vi "MotorControlMina.vi"() -> ()   [LabVIEW 2014]
uses:
  <vilib>/Utility/error.llb/DialogType.ctl
  <vilib>/Analysis/baseanly.llb/Mean (DBL).vi
  <vilib>/DAQmx/create/channels.llb/DAQmx Create Channel (DO-Digital Output).vi
  <vilib>/DAQmx/read.llb/DAQmx Read (Digital Bool 1Line 1Point).vi
  <vilib>/Utility/inputDevices.llb/joystickAcquire.vi
  <vilib>/Utility/inputDevices.llb/closeJoystick.vi
  <vilib>/DAQmx/create/channels.llb/DAQmx Create Channel (AI-Voltage-Basic).vi
  <vilib>/DAQmx/configure/timing.llb/DAQmx Timing (Sample Clock).vi
  <vilib>/DAQmx/read.llb/DAQmx Read (Analog 2D DBL NChan NSamp).vi
  <vilib>/DAQmx/create/channels.llb/DAQmx Create Channel (AO-Voltage-Basic).vi
  <vilib>/DAQmx/write.llb/DAQmx Write (Analog DBL 1Chan 1Samp).vi
  <vilib>/DAQmx/write.llb/DAQmx Write (Digital Bool 1Line 1Point).vi
  <vilib>/Analysis/NI_AALBase.lvlib
panel:
  in  "Offset (V)":dbl=5.0
  out "Oscillate Mirror? 2":bool
  out "Mirror Voltage":dbl
  in  "Oscillate Mirror?":bool
  in  "Period (s)":i32=1
  in  "Amplitude (V)":dbl=4.0
  in  "Stop":bool
  in  "ForceExtInitConst":dbl[](array[numeric])
  out "InstrumentMode":T1(ring)=enum."Shutdown"
  in  "XMotorRef":refnum<k7>(container)
  in  "YMotorRef":refnum<k7>(container)
  in  "ZMotorRef":refnum<k7>(container)
  out "JoystOffset":T2={"XOffset"=-99999, "YOffset"=-99999, "ZOffset"=-99999}
  out "RelJoyPos":T3
  in  "InterfaceSelector":T4(tab)
  in  "GoToTopDisp":bool
  in  "GoToBottDisp":bool
  in  "GoToExpLoc":bool
  in  "SaveTopDisp":bool
  in  "SaveBottDisp":bool
  in  "SaveExpLoc":bool
  out "Top Dispenser":T5={"X Pos (mm)"=0.5532008, "Y Pos (mm)"=0.030929338, "Z Pos (mm)"=0.77973413} {"Y Pos (mm)" format="%.3f"; "Z Pos (mm)" format="%.3f"; "X Pos (mm)" format="%.3f"}
  out "Bottom Dispenser":T5={"X Pos (mm)"=0.600309, "Y Pos (mm)"=-1.1540928, "Z Pos (mm)"=0.7938141} {"Y Pos (mm)" format="%.3f"; "Z Pos (mm)" format="%.3f"; "X Pos (mm)" format="%.3f"}
  out "Experiment Region":T5={"X Pos (mm)"=1.4278219, "Y Pos (mm)"=-0.74810517, "Z Pos (mm)"=0.7938141} {"Y Pos (mm)" format="%.3f"; "Z Pos (mm)" format="%.3f"; "X Pos (mm)" format="%.3f"}
  in  "PreviewPanel":T6(tab)
  out "Diagnostic Display":cluster{dbl, dbl}(graph)={100.78259213882863, 10.649843481998925}
  out "VertReading":dbl=0.0051513671875 format="%.3f"
  out "HorizReading":dbl=0.00535888671875 format="%.3f"
  out "QPD B \n(Steerable Trap)":T7={"Horizontal Voltage (V)"=-0.009930419921875, "Vertical Voltage (V)"=-0.077978515625, "Sum Voltage (V)"=-0.056793212890625, "Horizontal Signal (NormV)"=0.17485222998387961, "Vertical Signal (NormV)"=1.3730252552391187} {"Vertical Signal (NormV)" format="%.4f"; "Horizontal Signal (NormV)" format="%#.4f"; "Sum Voltage (V)" format="%.4f"; "Vertical Voltage (V)" format="%.4f"; "Horizontal Voltage (V)" format="%.4f"}
  out "QPD A \n(Fixed Trap)":T7={"Horizontal Voltage (V)"=-0.151220703125, "Vertical Voltage (V)"=-0.02420654296875, "Sum Voltage (V)"=-0.1012939453125, "Horizontal Signal (NormV)"=1.4928898529766208, "Vertical Signal (NormV)"=0.23897324656543747} {"Vertical Signal (NormV)" format="%.4f"; "Horizontal Signal (NormV)" format="%.4f"; "Sum Voltage (V)" format="%.4f"; "Vertical Voltage (V)" format="%.4f"; "Horizontal Voltage (V)" format="%.4f"}
  in  "PreviewDataAcquision":T8={"Sampling Freq (Hz)"=2500.0, "#Samples Averaged"=50}
  in  "Trap A (Steerable)  Params":T9={"X Stiff. (pN/nm)"=0.056, "X Alpha (nm/NV)"=976.0, "X Offset (NV)"=-0.02, "Y Stiff. (pN/nm)"=0.056, "Y Alpha (nm/NV)"=976.0, "Y Offset (NV)"=0.008}
  in  "Trap B (Fixed)  Params":T9={"X Stiff. (pN/nm)"=0.063, "X Alpha (nm/NV)"=1056.0, "X Offset (NV)"=-0.022, "Y Stiff. (pN/nm)"=0.063, "Y Alpha (nm/NV)"=1056.0, "Y Offset (NV)"=-0.013}
  in  "Z Motor Settings":T10={"Joyst Min Signal"=10.0, "Joyst Max Signal"=30000.0, "Vmax (mm/s)"=0.005, "Acc (mm/s/s)"=0.2, "+ JoystDirection"=2, "- JoystDirection"=1} {"Acc (mm/s/s)" format="%#.3f"; "Vmax (mm/s)" format="%#.3f"}
  in  "Y Motor Settings":T10={"Joyst Min Signal"=10.0, "Joyst Max Signal"=20000.0, "Vmax (mm/s)"=0.03, "Acc (mm/s/s)"=0.5, "+ JoystDirection"=1, "- JoystDirection"=2} {"Acc (mm/s/s)" format="%#.3f"; "Vmax (mm/s)" format="%#.3f"}
  in  "X Motor Settings":T10={"Joyst Min Signal"=10.0, "Joyst Max Signal"=20000.0, "Vmax (mm/s)"=0.03, "Acc (mm/s/s)"=0.5, "+ JoystDirection"=2, "- JoystDirection"=1} {"Acc (mm/s/s)" format="%#.3f"; "Vmax (mm/s)" format="%#.3f"}
  in  "Motor Cruise Param":T11={"X Acc (mm/s^2)"=0.3, "X Vmax (mm/s)"=0.3, "Y Acc (mm/s^2)"=0.3, "Y Vmax (mm/s)"=0.3, "Z Acc (mm/s^2)"=0.1, "Z Vmax (mm/s)"=0.1}
  in  "Motor Limits":T12={"XMin"=-0.8, "XMax"=3.0, "YMin"=-2.0, "YMax"=2.0, "ZMin"=0.0, "ZMax"=2.0}
  in  "Steerable Mirror Calibration":T13={"Hor. Scaling (nm/V)"=760.0, "Vert. Scaling (nm/V)"=760.0, "Hor. Mirr. Offset (V)"=0.0, "Vert. Mirr. Offset (V)"=0.0}
  in  "SampRate/Ch":dbl=25000.0
  in  "AveragingWindow":i32=10
  in  "Steerable \nTrap\n(F12)":bool
  in  "Fixed\nTrap\n(F11)":bool
  in  "BMHorizSlider(V)":dbl(slide)=0.0059356689453125 scale=0.0..10.0
  in  "BMSliderVert(V)":dbl(slide)=0.005126953125 scale=0.0..10.0 scale format="%#_3f"
  in  "Align Traps Vertically":bool
  in  "MaxHorizontalTrapSeparation":bool
  out "X Motor State":T14={"Direction"=0, "Vel (mm/s)"=0.0, "IsActive?"=FALSE, "Pos (mm)"=-0.2957381} {"Pos (mm)" format="%#.3f"; "Vel (mm/s)" format="%#.4f"}
  out "Y Motor State":T14={"Direction"=0, "Vel (mm/s)"=0.0, "IsActive?"=FALSE, "Pos (mm)"=0.016441232} {"Pos (mm)" format="%#.3f"; "Vel (mm/s)" format="%#.4f"}
  out "Z Motor State":T14={"Direction"=0, "Vel (mm/s)"=0.0, "IsActive?"=FALSE, "Pos (mm)"=-0.26253498} {"Pos (mm)" format="%#.3f"; "Vel (mm/s)" format="%#.4f"}
  out "Move Z":bool
  out "Move XY":bool
  in  "MotorLoopDelay":u32=100
  out "Waveform Chart":T15(graph)={"[0]"=0.0023651123, "[1]"=0.0025787354, "[2]"=0.0019226074, "[3]"=0.0018310547, "[4]"=0.006378174, "[5]"=0.004486084, "[6]"=0.0008239746, "[7]"=0.0034179688}
  in  "StopPassiveMode":bool caption="stop"
  out "LowFreqFilePath":string="C:\\Data\\091813\\091813N02.psv"
  in  "PMVertSlider(V)":dbl(slide)=0.005145263671875 scale=0.0..10.0 scale format="%#_3f"
  in  "PMHorizSlider(V)":dbl(slide)=0.0045623779296875 scale=2.0..10.0
  out "IsPassiveModeActive?":bool caption="stop"
  out "Force TrapA":cluster{"x":dbl[], "y":dbl[]}[](graph)
  out "Noise-Ext":cluster{"x":dbl[], "y":dbl[]}[](graph)
  out "Force TrapB":cluster{"x":dbl[], "y":dbl[]}[](graph)
  out "OffsetFilePath":string="C:\\Data\\091813\\091813N08.ofs"
  in  "InitialConst":dbl[](array[numeric])
  in  "Stop Voltage (V)":dbl=4.0
  out "OM Vert MTA Voltage":dbl=0.0042724609375 format="%#.3f"
  out "OM Horiz MTA Voltage":dbl format="%#.3f"
  in  "HorizMirrCalib(nm/V)":dbl=752.0
  in  "HorizMirrOffs(V)":dbl
  in  "ClearChart":bool
  in  "Step (V)":dbl=0.01
  in  "#PtsToWait":i32=100
  in  "VertMirrOffs(V)":dbl
  in  "VertMirrCalib(nm/V)":dbl=752.0
  out "IsOffsetModeActive?":bool caption="stop"
  in  "StopOffset":bool caption="stop"
  out "ProgressBar":i32(slide)=200 min=0 max=512 step=1 scale=0.0..200.0
  in  "WindowSample#":i32=2048
  out "HiFreqDiagnostic":T16(graph)={"[0]"=0.002342537045478821, "[1]"=0.0025282055139541626, "[2]"=0.0019662082195281982, "[3]"=0.0019291043281555176, "[4]"=0.005142837762832642, "[5]"=0.0045330822467803955, "[6]"=0.0008034706115722656, "[7]"=0.0034596025943756104}
  in  "HiFSamplingRate/Ch":dbl=25000.0
  out "File Name and Path":string="C:\\Data\\091813\\091813N01.brw"
  in  "Total#OfWindows":dbl=200.0
  out "IsForceExtActive?":bool=TRUE
  in  "FEX Axis":bool=TRUE
  out "ForceExtensionFilePath":string="C:\\Data\\091813\\091813N00.pul"
  in  "StopForceExtension":bool caption="stop"
  in  "#FEXPtsToWait":i32=500
  in  "Mirror Step (V)":dbl=0.0020000000949949026
  out "FEX Force TrapA":cluster{"x":dbl[], "y":dbl[]}[](graph)
  out "FEX Noise-Ext":cluster{"x":dbl[], "y":dbl[]}[](graph)
  in  "Direction":bool=TRUE
  in  "IsPullActive?":bool
  in  "Clear FEX Chart":bool
  in  "FEX HorizMirrOffs(V)":dbl
  in  "FEX HorizMirrCalib(nm/V)":dbl=752.0
  out "FEX Mirror Y Volt":dbl=0.00537109375 format="%#.3f"
  out "FEX Mirror X Volt":dbl=0.004638671875 format="%#.3f"
  # "ClpXP Optical Tweezers"
  # "Chamber Locations"
  # "Need a Button Here that would read the \nNormalized Offset and save it"
  # "Off"
  # "On"
  # "Off"
  # "On"
  # "Thorlabs Motor Status"
  # "Passive Mode"
  # "when I switch tabs from the passive mode to basic mode, the recording doesn't stop"
  # "The sliders don't do anything in passive mode, fix it"
  # "Whenever I click on Ackquire Offset, it goes back to the basic operation, then I have to ckick again"
  # "Trap Motion Control"
  # "Steerable Mirror Info"
  # "Zero-Force Offset Mode"
  # "High Frequency Data Acquisition"
  # "Adjust the length of acquisition time"
  # "Force-Extension Mode"
  # "Y"
  # "+"
  # "X"
  # "-"
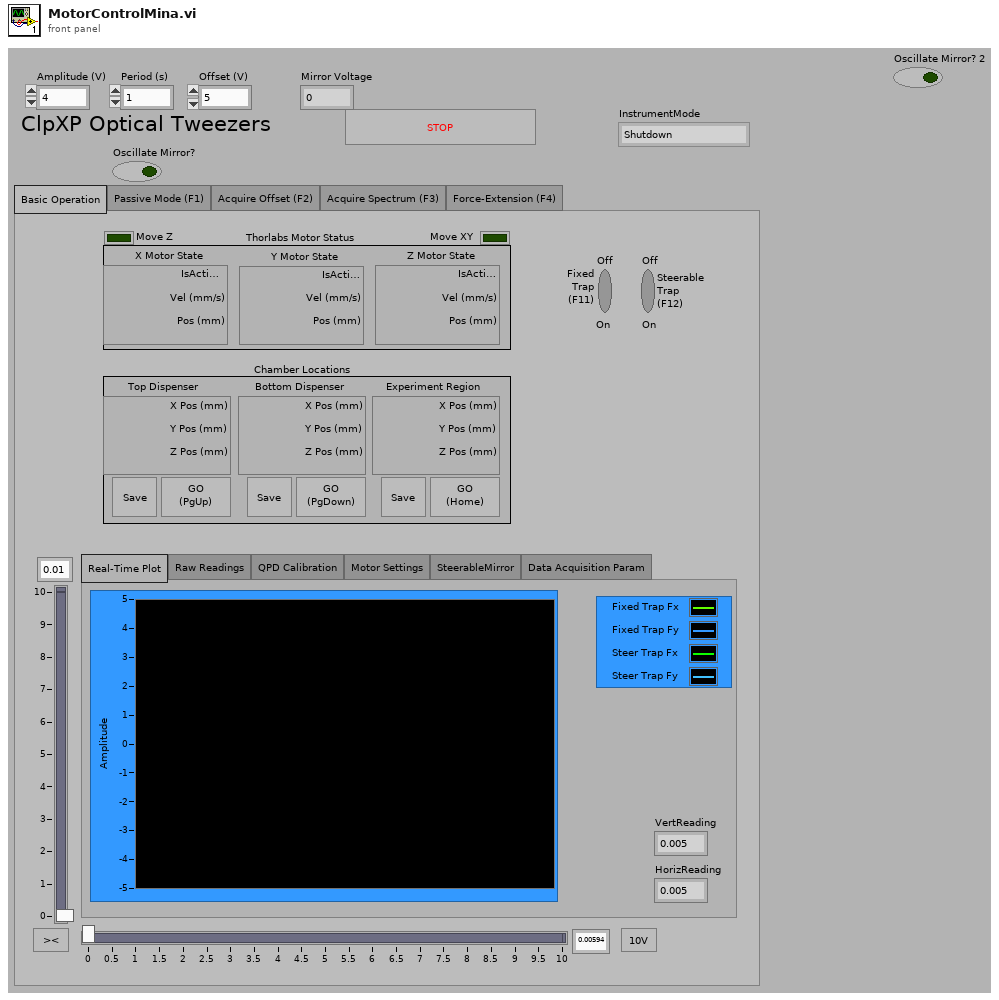
[diagram p1: front panel]
types:
  T1 = enum16{"InitializeJoystick", "InitializeMotors", "BasicMode", "PassiveMode", "AcquireOffsetMode", "AcquireSpectrumMode", "Force-ExtensionMode", "Shutdown"}
  T2 = cluster{"XOffset":i32, "YOffset":i32, "ZOffset":i32}
  T3 = cluster{"XRelPos":i32, "YRelPos":i32, "ZRelPos":i32}
  T4 = enum32{"Basic Operation", "Passive Mode (F1)", "Acquire Offset (F2)", "Acquire Spectrum (F3)", "Force-Extension (F4)"}
  T5 = cluster{"X Pos (mm)":sgl, "Y Pos (mm)":sgl, "Z Pos (mm)":sgl}
  T6 = enum32{"Real-Time Plot", "Raw Readings", "QPD Calibration", "Motor Settings", "SteerableMirror", "Data Acquisition Param"}
  T7 = cluster{"Horizontal Voltage (V)":dbl, "Vertical Voltage (V)":dbl, "Sum Voltage (V)":dbl, "Horizontal Signal (NormV)":dbl, "Vertical Signal (NormV)":dbl}
  T8 = cluster{"Sampling Freq (Hz)":dbl, "#Samples Averaged":i32}
  T9 = cluster{"X Stiff. (pN/nm)":dbl, "X Alpha (nm/NV)":dbl, "X Offset (NV)":dbl, "Y Stiff. (pN/nm)":dbl, "Y Alpha (nm/NV)":dbl, "Y Offset (NV)":dbl}
  T10 = cluster{"Joyst Min Signal":dbl, "Joyst Max Signal":dbl, "Vmax (mm/s)":sgl, "Acc (mm/s/s)":sgl, "+ JoystDirection":i32, "- JoystDirection":i32}
  T11 = cluster{"X Acc (mm/s^2)":sgl, "X Vmax (mm/s)":sgl, "Y Acc (mm/s^2)":sgl, "Y Vmax (mm/s)":sgl, "Z Acc (mm/s^2)":sgl, "Z Vmax (mm/s)":sgl}
  T12 = cluster{"XMin":sgl, "XMax":sgl, "YMin":sgl, "YMax":sgl, "ZMin":sgl, "ZMax":sgl}
  T13 = cluster{"Hor. Scaling (nm/V)":dbl, "Vert. Scaling (nm/V)":dbl, "Hor. Mirr. Offset (V)":dbl, "Vert. Mirr. Offset (V)":dbl}
  T14 = cluster{"Direction":i32, "Vel (mm/s)":sgl, "IsActive?":bool, "Pos (mm)":sgl}
  T15 = cluster{"[0]":sgl, "[1]":sgl, "[2]":sgl, "[3]":sgl, "[4]":sgl, "[5]":sgl, "[6]":sgl, "[7]":sgl}
  T16 = cluster{"[0]":dbl, "[1]":dbl, "[2]":dbl, "[3]":dbl, "[4]":dbl, "[5]":dbl, "[6]":dbl, "[7]":dbl}
  T17 = typedef "DialogType.ctl" = u16
  T18 = cluster{"XMotorRef":refnum<k7>, "YMotorRef":refnum<k7>, "ZMotorRef":refnum<k7>}
  T19 = enum16{"open", "open or create", "create or replace", "create", "open (read only)"}
  T20 = cluster{"[0]":dbl, "[1]":dbl, "[2]":dbl, "[3]":dbl, "[4]":dbl, "[5]":dbl, "[6]":dbl, "[7]":dbl}[]
  T21 = cluster{"AI0: Vy Steer Trap":dbl, "AI1: Vy Fixed Trap":dbl, "AI2: Vx Steer Trap":dbl, "AI3: Vx Fixed Trap":dbl, "AI4: MTA Yaxis":dbl, "AI5: MTA Xaxis":dbl, "AI6: Vsum Steer Trap":dbl, "AI7: Vsum Fixed Trap":dbl}
  T22 = cluster{"Fx Fixed Trap":dbl, "Fy Fixed Trap":dbl, "Fx Steerable Trap":dbl, "Fy Steerable Trap":dbl}
  T23 = cluster{"Fx Fixed Trap":dbl, "Fx Steerable Trap":dbl}
  T24 = cluster{"Steerable \nTrap\n(F12)":refnum<vi>, "Fixed\nTrap\n(F11)":refnum<vi>}
  T25 = cluster{"Motor Reference":refnum<k7>, "Motor Reference":refnum<k7>, "Motor Reference":refnum<k7>}
  T26 = cluster{"X axis":i32, "Y axis":i32, "Z axis":i32, "X axis rotation":i32, "Y axis rotation":i32, "Z axis rotation":i32, "U axis":i32, "V axis":i32}
  T27 = cluster{"button 1":bool, "button 2":bool, "button 3":bool, "button 4":bool, "button 5":bool, "button 6":bool, "button 7":bool, "button 8":bool, "button 9":bool, "button 10":bool, "button 11":bool, "button 12":bool, "button 13":bool, "button 14":bool, "button 15":bool, "button 16":bool, "button 17":bool, "button 18":bool, "button 19":bool, "button 20":bool, "button 21":bool, "button 22":bool, "button 23":bool, "button 24":bool, "button 25":bool, "button 26":bool, "button 27":bool, "button 28":bool, "button 29":bool, "button 30":bool, "button 31":bool, "button 32":bool}
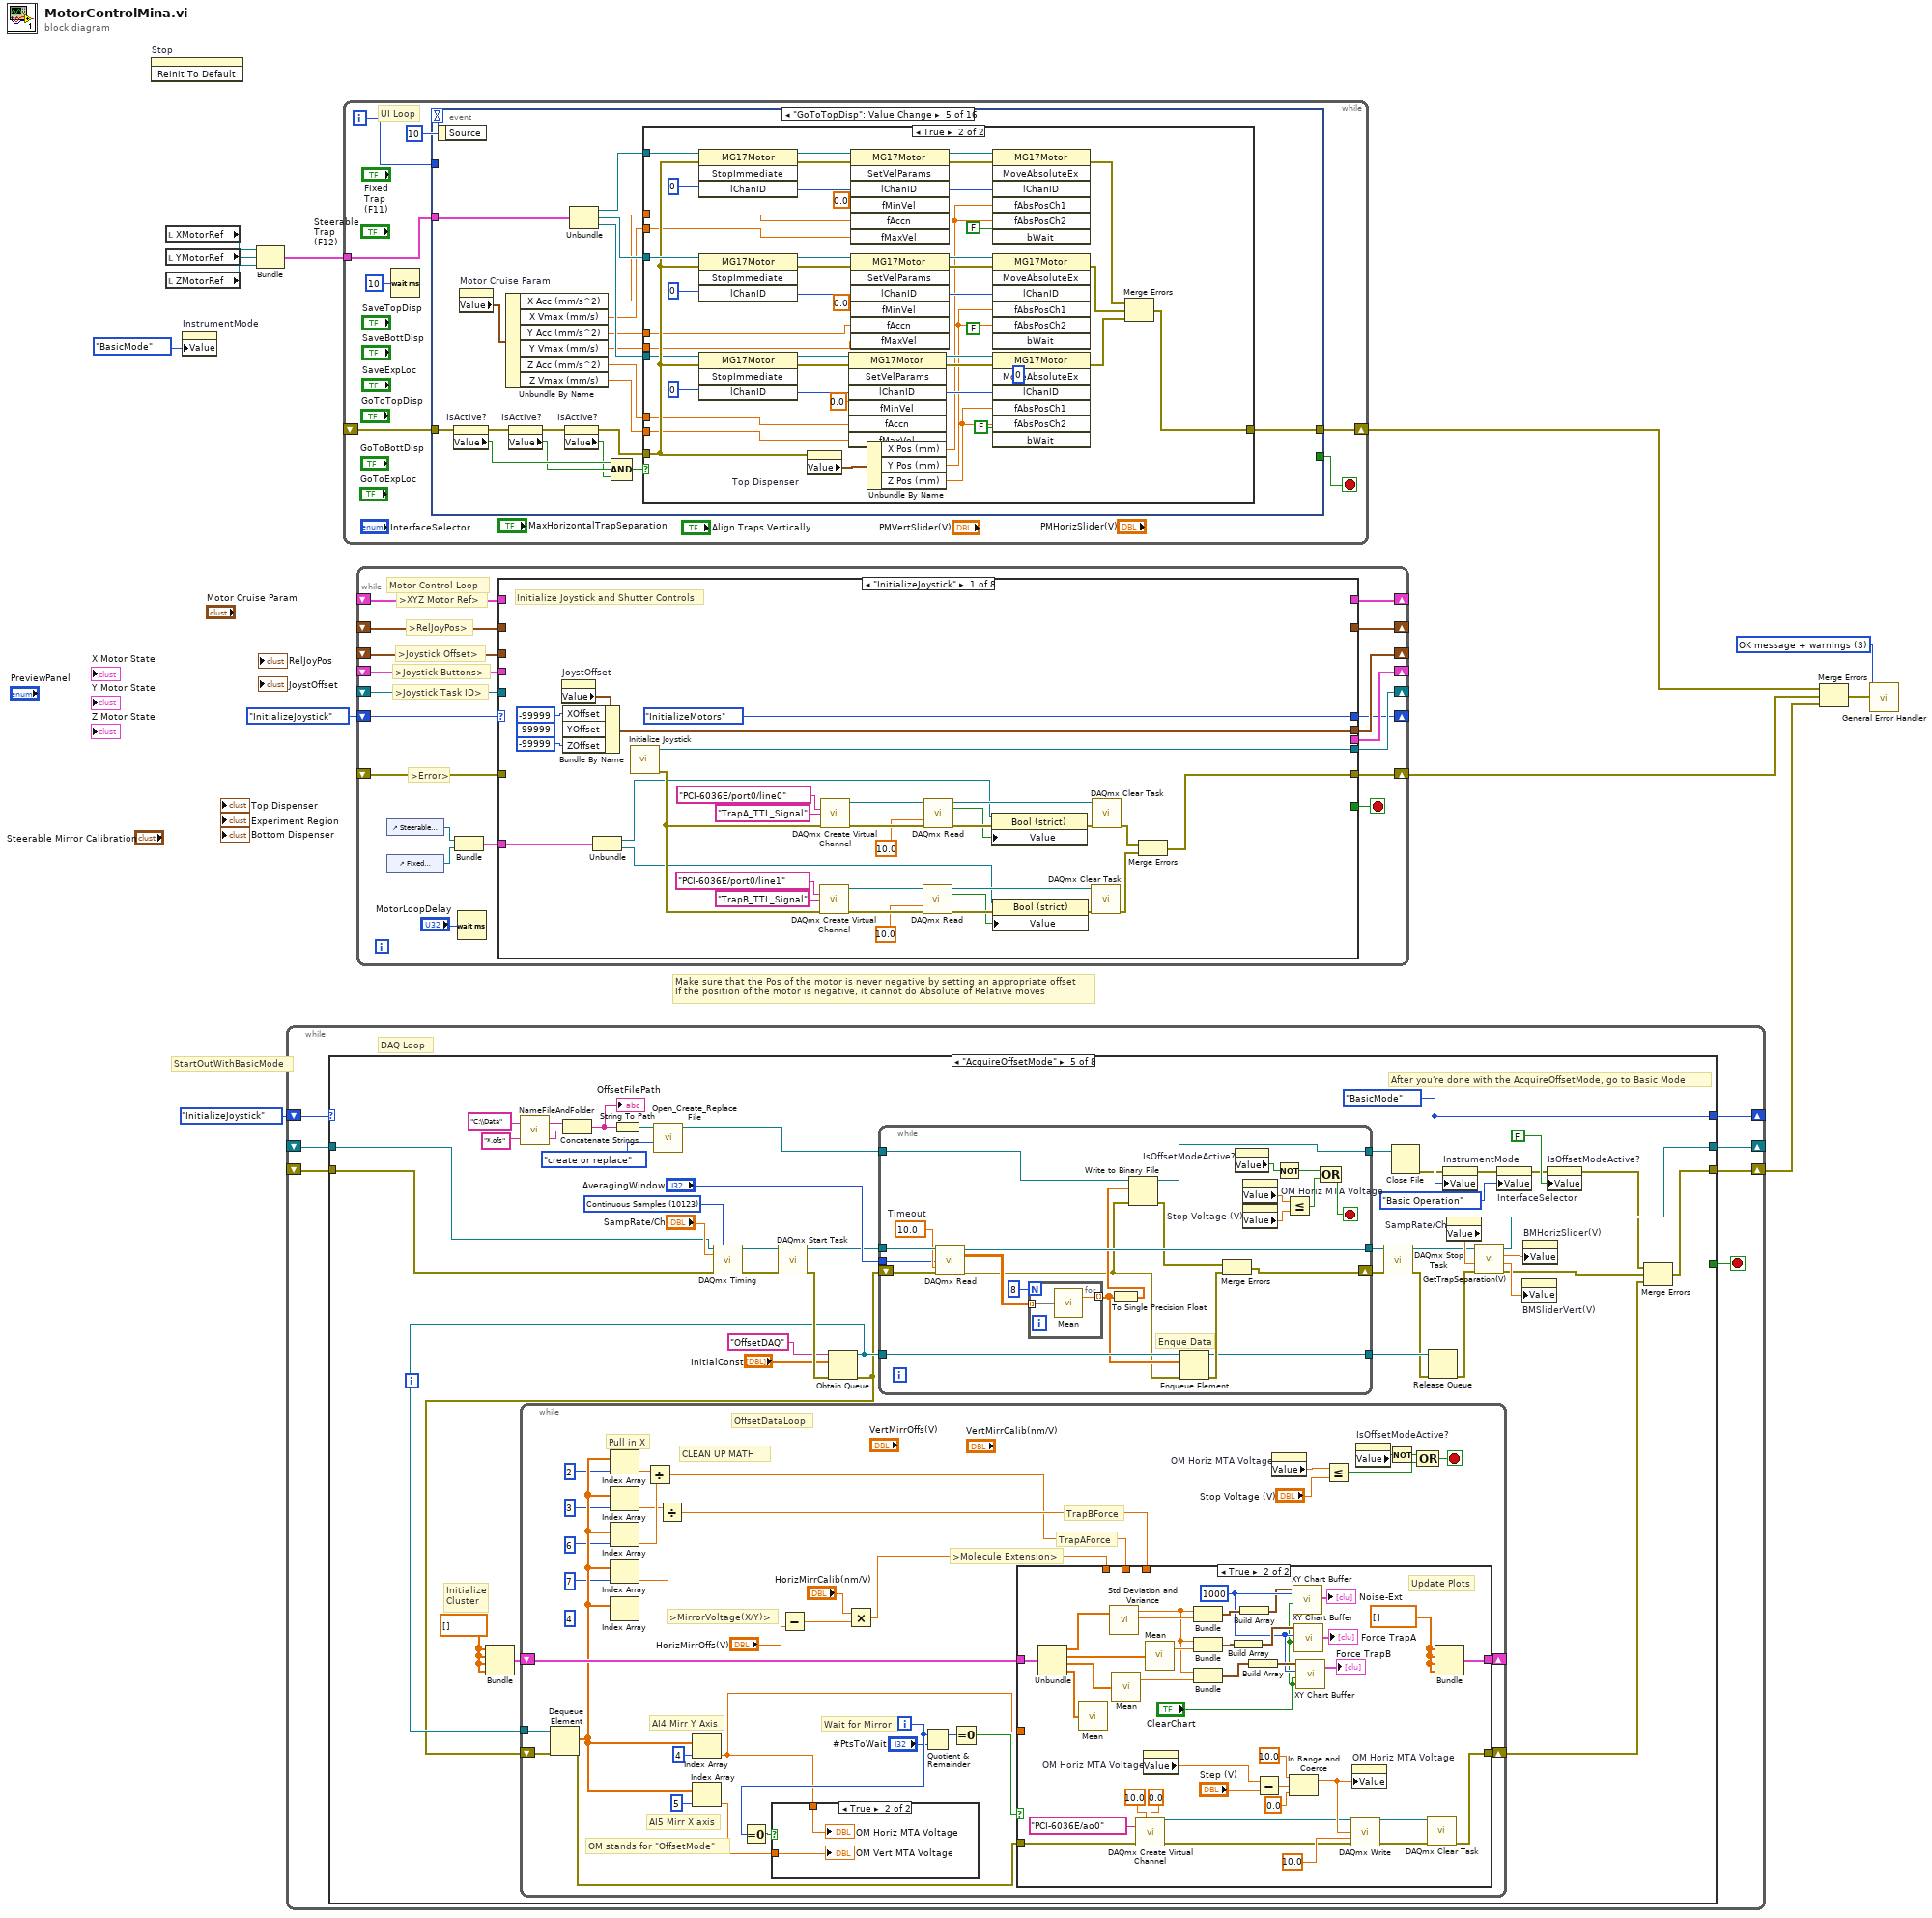
[diagram p0: block diagram]
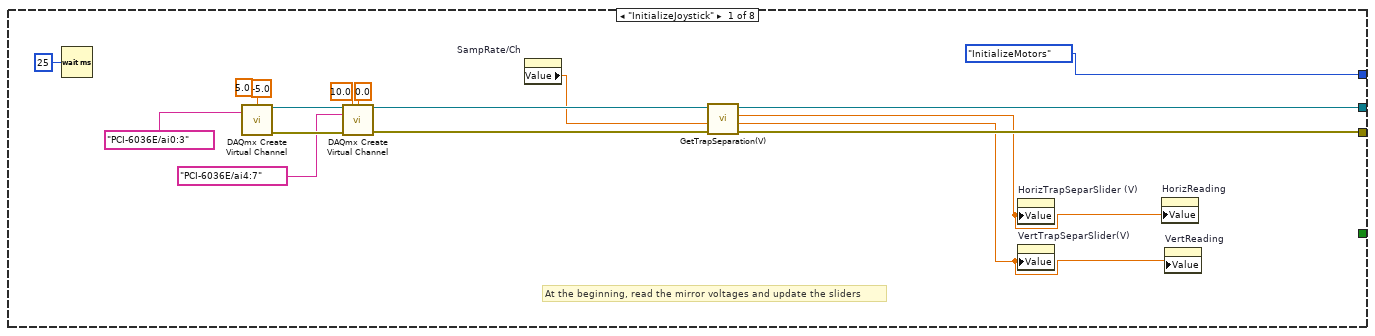
[diagram p2: hidden frame]
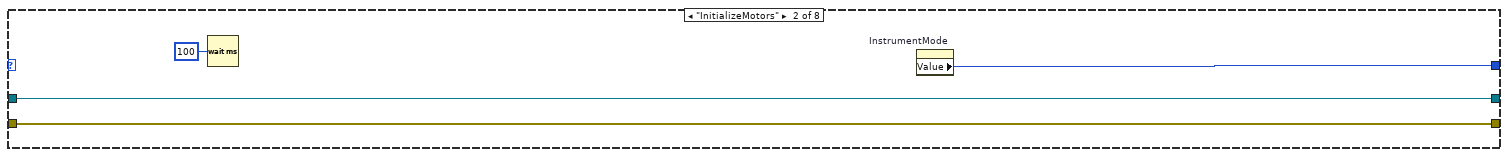
[diagram p3: hidden frame]
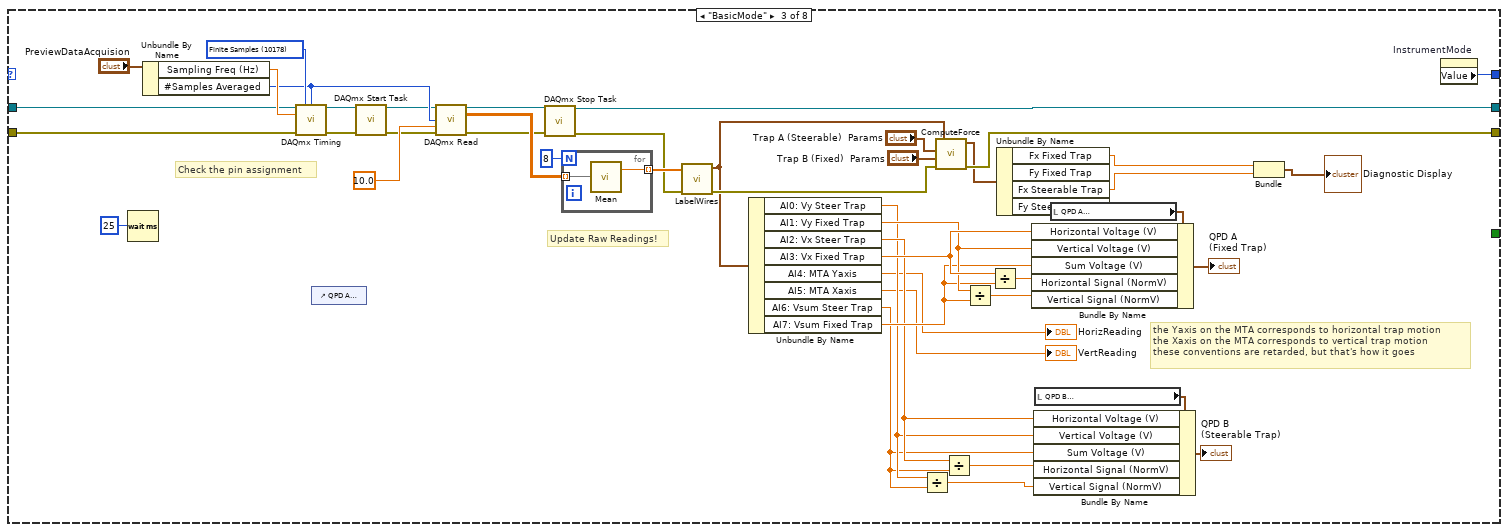
[diagram p4: hidden frame]
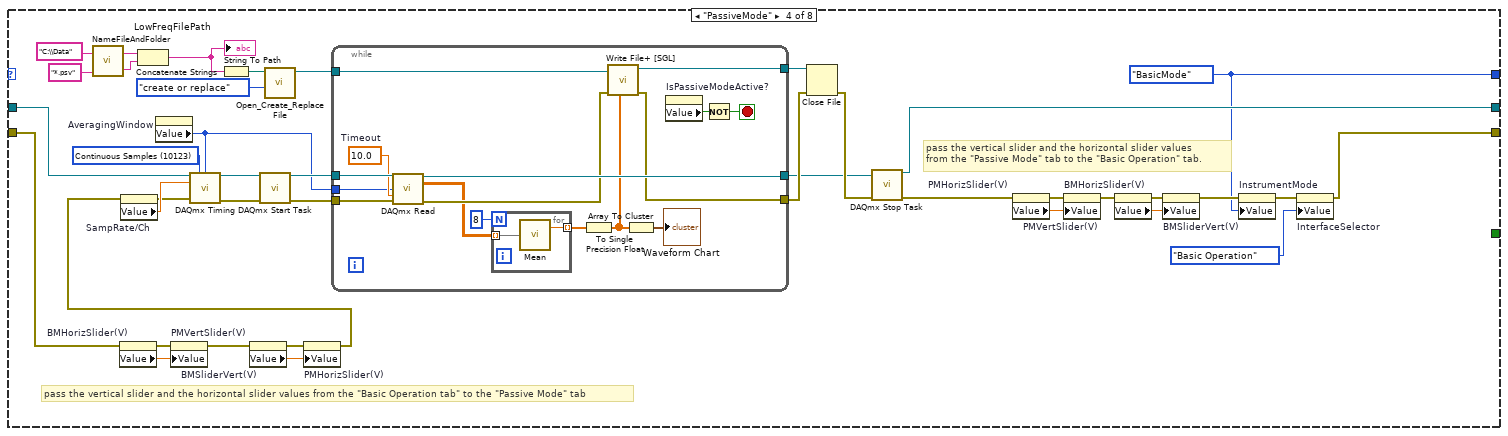
[diagram p5: hidden frame]
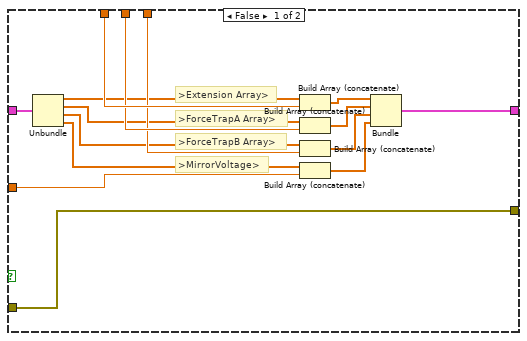
[diagram p7: hidden frame]
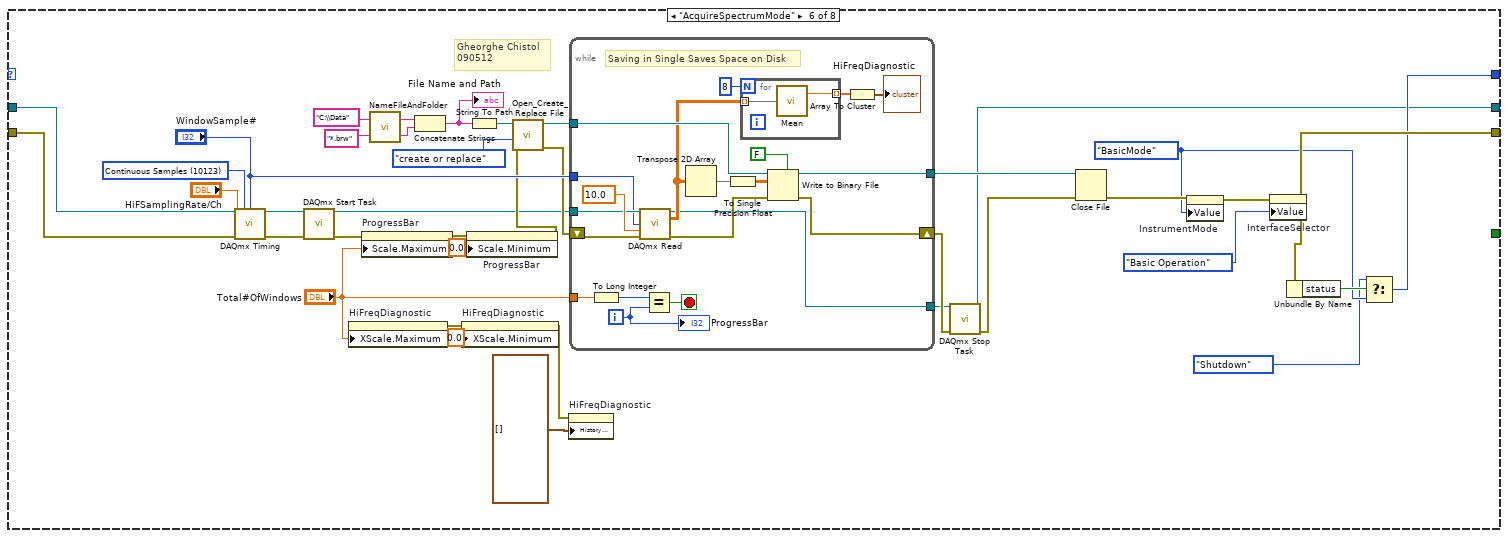
[diagram p8: hidden frame]
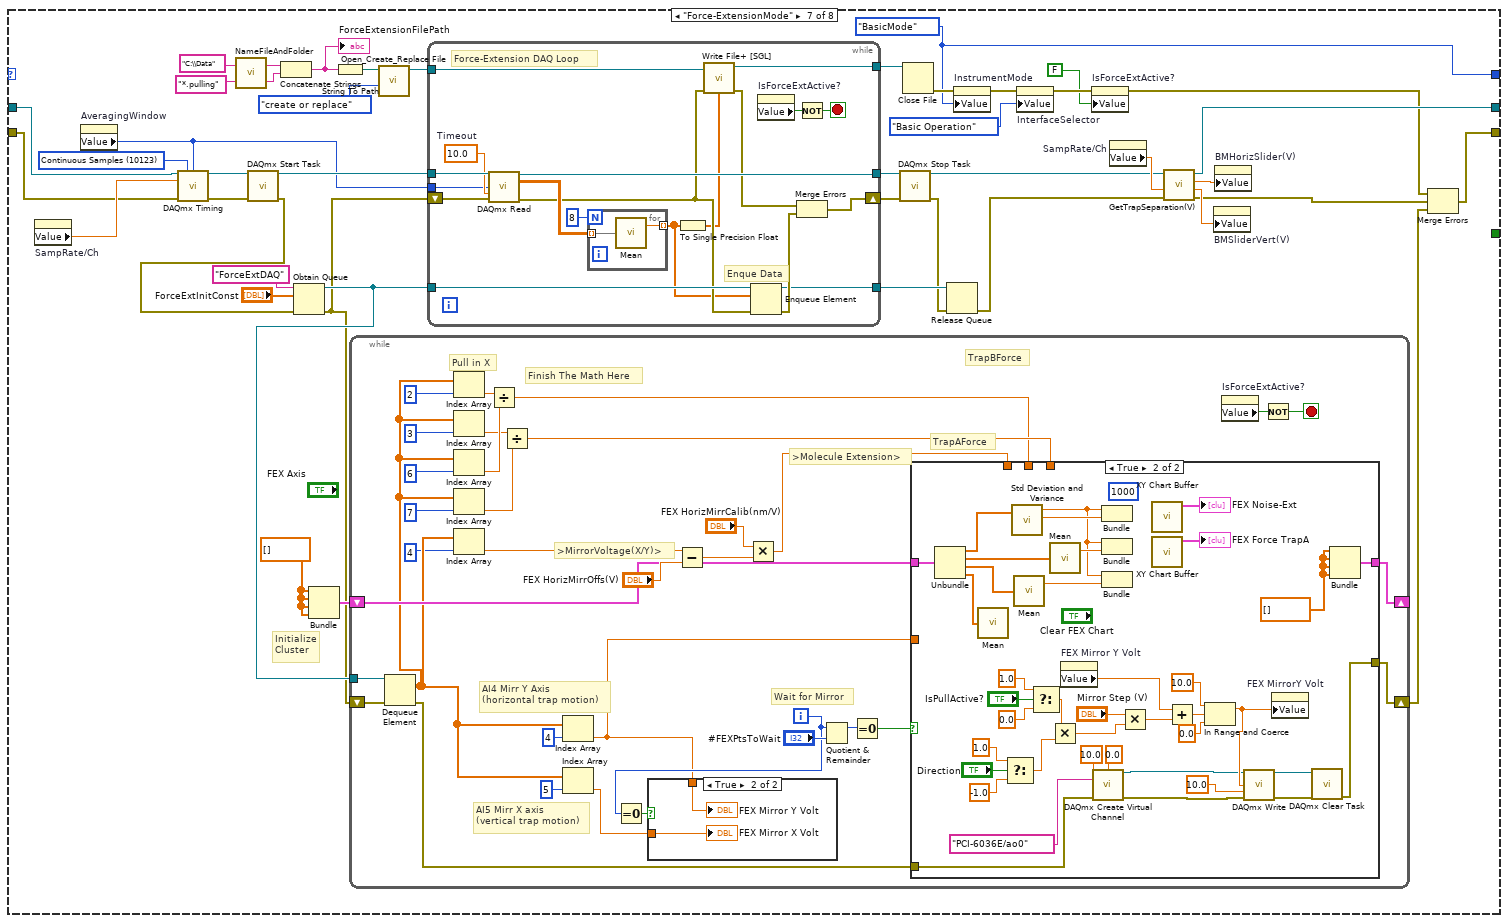
[diagram p9: hidden frame]
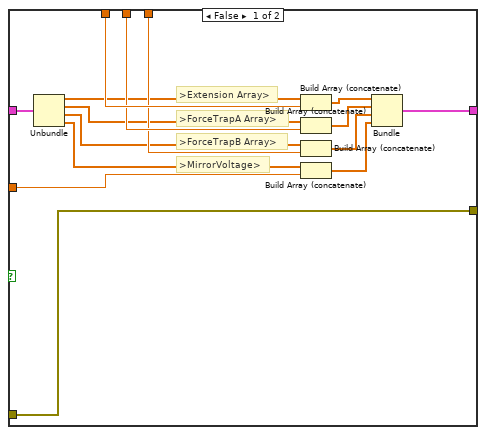
[diagram p11: hidden frame]
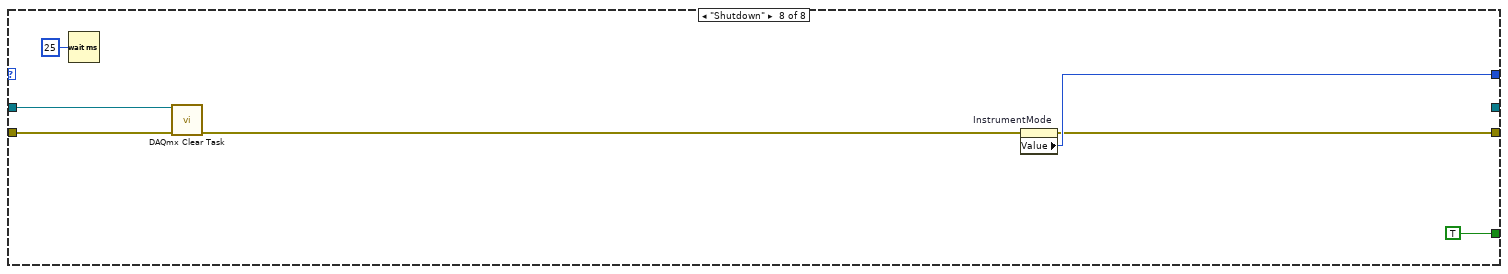
[diagram p12: hidden frame]
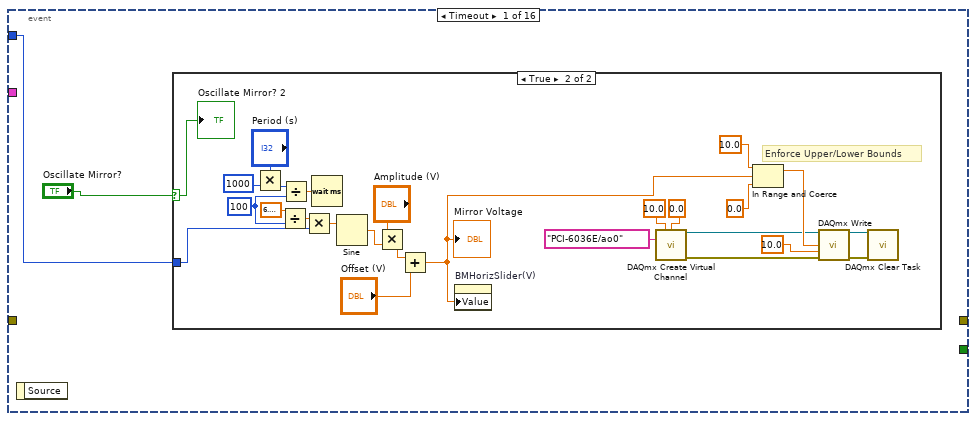
[diagram p13: hidden frame]
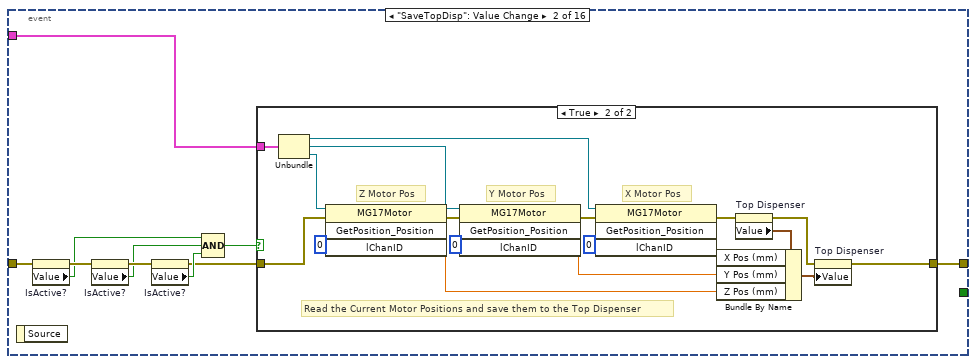
[diagram p15: hidden frame]
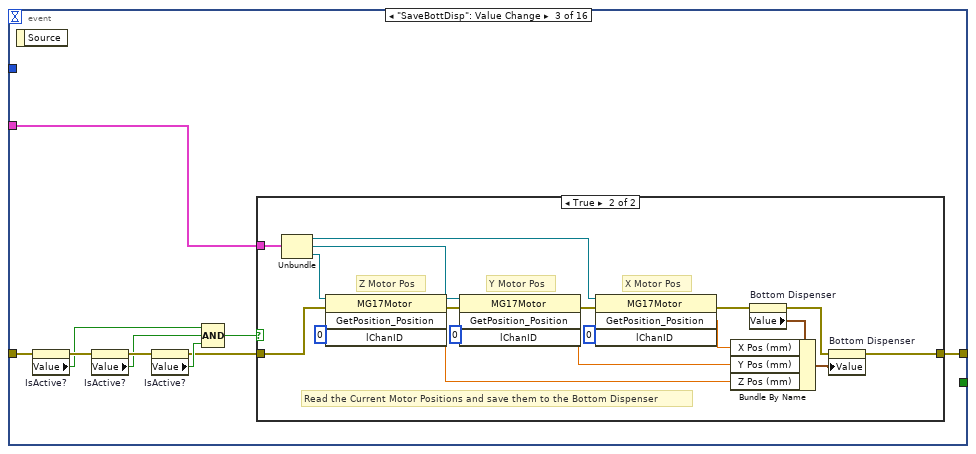
[diagram p17: hidden frame]
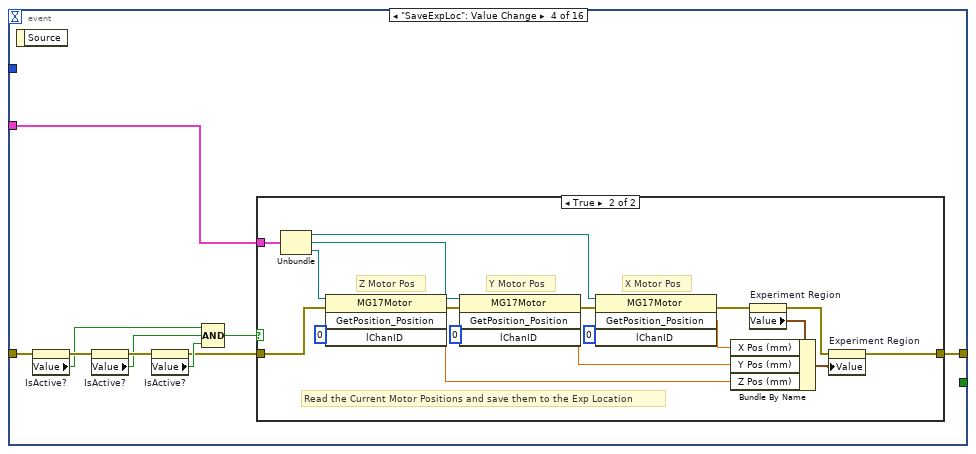
[diagram p19: hidden frame]
diagram:
  w2 = T17 3 items=["no dialog", "OK message", "continue or stop message", "OK message + warnings", "continue/stop + warnings"] ("type of dialog (OK msg:1)")
  # "StartOutWithBasicMode"
  # "Make sure that the Pos of the motor is never negative by setting an appropriate offset\nIf the position of the motor is negative, it cannot do Absolute of Relative moves"
  n1 = invoke on="Stop" class="Bool" method="Reinit To Default"() -> ()  [unwired: 3 in, 3 out]
  n2 = local read "XMotorRef"() -> (w12:refnum<k7>)
  n3 = local read "YMotorRef"() -> (w11:refnum<k7>)
  n4 = local read "ZMotorRef"() -> (w10:refnum<k7>)
  n5 = property on="InstrumentMode" class="Enum (strict)"("Value"=T1."BasicMode") -> ()  [unwired: 2 in, 2 out]
  n6 = Bundle("XMotorRef"=w12, "YMotorRef"=w11, "ZMotorRef"=w10) -> (w9:T18)  [unwired: 1 in]
  n7 = while {
    shift-right: [w14] -> _
    shift-left: T1."InitializeJoystick" ("Value") -> [w15]
    shift-right: [w17] -> w7
    shift-left: _ -> [w18]
    shift-right: [w13] -> _
    shift-left: _ -> [w19]
    stop <- w16 stop-if-true
    # "DAQ Loop"
    n8 = case shown="\"AcquireOffsetMode\"" w15 {
      tunnel: w19 -> [_ w37 w67 w109 w157 w308 w382 w523]
      tunnel: w18 -> [_ w36 w79 w100 w170 w327 w390 w526]
      tunnel: [w23 w36 w49 w87 w145 w322 w369 w524] -> w17
      tunnel: [_ _ _ _ _ _ _ TRUE] -> w16
      tunnel: [T1."InitializeMotors" ("Value") w38 w77 w88 w162 w318 w379 w528] -> w14
      tunnel: [w24 w37 w66 w106 w150 w307 w373 _] -> w13
      frame "InitializeJoystick" {
        (unwired) 5.0 ("Maximum Value")
        # "At the beginning, read the mirror voltages and update the sliders"
        n9 = Wait (ms)(milliseconds to wait=u32 25) -> ()  [unwired: 1 out]
        n10 = call-poly <vilib>:"DAQmx Create Virtual Channel.vi"("minimum value"=-5.0 ("Minimum Value"), "physical channels"=tag "PCI-6036E/ai0:3" ("Physical Channel")) -> ("task out"=w32:refnum<k21>, "error out"=w31:errorcluster)  [unwired: 12 in]
        n11 = call-poly <vilib>:"DAQmx Create Virtual Channel.vi"("task in"=w32, "maximum value"=10.0, "minimum value"=0.0, "physical channels"=tag "PCI-6036E/ai4:7", "error in"=w31) -> ("task out"=w27:refnum<k21>, "error out"=w26:errorcluster)  [unwired: 9 in]
        n12 = property on="SampRate/Ch" class="DigNum (strict)"() -> ("Value"=w25:dbl)  [unwired: 2 in, 2 out]
        n13 = call "GetTrapSeparation(V).vi"("ErrorIn"=w26, "AcquisitionRatePerChannel"=w25, "DAQ Task"=w27) -> ("ErrorOut"=w23:errorcluster, "VertTrapSeparation(V)"=w21:dbl, "HorTrapSeparation(V)"=w22:dbl, "DAQ Task"=w24:refnum<k21>)  [unwired: 1 in]
        n14 = property on="HorizTrapSeparSlider (V)" class="Slide (strict)"("Value"=w22) -> ()  [unwired: 2 in, 2 out]
        n15 = property on="VertTrapSeparSlider(V)" class="Slide (strict)"("Value"=w21) -> ()  [unwired: 2 in, 2 out]
        n16 = property on="HorizReading" class="DigNum (strict)"("Value"=w22) -> ()  [unwired: 2 in, 2 out]
        n17 = property on="VertReading" class="DigNum (strict)"("Value"=w21) -> ()  [unwired: 2 in, 2 out]
      }
      frame "InitializeMotors" {
        n18 = Wait (ms)(milliseconds to wait=u32 100) -> ()  [unwired: 1 out]
        n19 = property on="InstrumentMode" class="Enum (strict)"() -> ("Value"=w38:T1)  [unwired: 2 in, 2 out]
      }
      frame "BasicMode" {
        w78 = 10178 items=["Finite Samples"=10178, "Continuous Samples"=10123, "Hardware Timed Single Point"=12522] ("sample mode")
        # "the Yaxis on the MTA corresponds to horizontal trap motion\nthe Xaxis on the MTA corresponds to vertical trap motion\nthese conventions are retarded, but that's how it goes"
        # "Update Raw Readings!"
        # "Check the pin assignment"
        n20 = Wait (ms)(milliseconds to wait=u32 25) -> ()  [unwired: 1 out]
        n21 = Unbundle By Name("PreviewDataAcquision") -> ("Sampling Freq (Hz)"=w82:dbl, "#Samples Averaged"=w76:i32)
        n22 = call-poly <vilib>:"DAQmx Timing.vi"("task/channels in"=w67, "sample mode"=w78, "samples per channel"=w76, "rate"=w82, "error in"=w79) -> ("task out"=w74:refnum<k21>, "error out"=w73:errorcluster)  [unwired: 9 in]
        n23 = control-ref of="QPD A \n(Fixed Trap)"() -> ()  [unwired: 1 out]
        n24 = call <vilib>:"DAQmx Start Task.vi"("task/channels in"=w74, "error in"=w73) -> ("task out"=w72:refnum<k21>, "error out"=w71:errorcluster)  [unwired: 12 in]
        n25 = call-poly <vilib>:"DAQmx Read.vi"("task/channels in"=w72, "number of samples per channel"=w76, "timeout"=10.0, "error in"=w71) -> ("task out"=w70:refnum<k21>, "data"=w84:dbl[][], "error out"=w69:errorcluster)  [unwired: 9 in]
        n26 = call <vilib>:"DAQmx Stop Task.vi"("task/channels in"=w70, "error in"=w69) -> ("task out"=w66:refnum<k21>, "error out"=w65:errorcluster)  [unwired: 12 in]
        n27 = for {
          N: 8 -> [_]
          tunnel: w84 -> [w86] mode=indexing
          tunnel: [w85] -> w68 mode=indexing
          n28 = call-poly <vilib>:"Mean.vi"("X"=w86) -> ("mean"=w85:dbl)  [unwired: 1 out]
        }
        n29 = call "LabelWires.vi"("Error In"=w65, "DAQ Raw Measurement Array"=w68) -> ("Error Out"=w50:errorcluster, "Named DAQ Cluster"=w40:T21)  [unwired: 4 in]
        n30 = Unbundle By Name(w40) -> ("AI0: Vy Steer Trap"=w55:dbl, "AI1: Vy Fixed Trap"=w59:dbl, "AI2: Vx Steer Trap"=w56:dbl, "AI3: Vx Fixed Trap"=w60:dbl, "AI4: MTA Yaxis"=→"HorizReading":dbl, "AI5: MTA Xaxis"=→"VertReading":dbl, "AI6: Vsum Steer Trap"=w54:dbl, "AI7: Vsum Fixed Trap"=w58:dbl)
        n31 = Divide(x=w55, y=w54) -> (x/y=w53:dbl)
        n32 = call "ComputeForce.vi"("Error In"=w50, "Fixed Trap Params"="Trap B (Fixed)  Params", "Steerable Trap Params"="Trap A (Steerable)  Params", "Named DAQ Cluster"=w40) -> ("Error Out"=w49:errorcluster, "Computed Forces"=w44:T22)  [unwired: 2 out]
        n33 = Divide(x=w56, y=w54) -> (x/y=w45:dbl)
        n34 = Divide(x=w59, y=w58) -> (x/y=w57:dbl)
        n35 = Divide(x=w60, y=w58) -> (x/y=w46:dbl)
        n36 = Unbundle By Name(w44) -> ("Fx Fixed Trap"=w43:dbl, "Fx Steerable Trap"=w42:dbl)  [unwired: 2 out]
        n37 = local read "QPD B \n(Steerable Trap)"() -> (w62:T7)
        n38 = Bundle By Name(cluster=w62, "Horizontal Voltage (V)"=w56, "Vertical Voltage (V)"=w55, "Sum Voltage (V)"=w54, "Horizontal Signal (NormV)"=w45, "Vertical Signal (NormV)"=w53) -> (→"QPD B \n(Steerable Trap)":T7)
        n39 = local read "QPD A \n(Fixed Trap)"() -> (w64:T7)
        n40 = Bundle By Name(cluster=w64, "Horizontal Voltage (V)"=w60, "Vertical Voltage (V)"=w59, "Sum Voltage (V)"=w58, "Horizontal Signal (NormV)"=w46, "Vertical Signal (NormV)"=w57) -> (→"QPD A \n(Fixed Trap)":T7)
        n41 = Bundle("Fx Fixed Trap"=w43, "Fx Steerable Trap"=w42) -> (→"Diagnostic Display":T23)  [unwired: 1 in]
        n42 = property on="InstrumentMode" class="Enum (strict)"() -> ("Value"=w77:T1)  [unwired: 2 in, 2 out]
      }
      frame "PassiveMode" {
        w88 = T1."BasicMode" ("Value")
        w113 = 10123 items=["Finite Samples"=10178, "Continuous Samples"=10123] ("sample mode")
        # "pass the vertical slider and the horizontal slider values \nfrom the \"Passive Mode\" tab to the \"Basic Operation\" tab."
        # "pass the vertical slider and the horizontal slider values from the \"Basic Operation tab\" to the \"Passive Mode\" tab"
        n43 = call "NameFileAndFolder.vi"("ext"="*.psv", "Head Directory"="C:\\Data" ("path")) -> ("New Filename"=w123:string, "Sub Directory"=w124:string)
        n44 = property on="BMHorizSlider(V)" class="Slide (strict)"(error in=w100) -> (error out=w103:errorcluster, "Value"=w105:dbl)  [unwired: 1 in, 1 out]
        n45 = Concatenate Strings(w124, w123) -> (w120:string)
        "LowFreqFilePath" <- w120
        n46 = property on="AveragingWindow" class="DigNum (strict)"() -> ("Value"=w108:i32)  [unwired: 2 in, 2 out]
        n47 = property on="PMVertSlider(V)" class="Slide (strict)"(error in=w103, "Value"=w105) -> (error out=w102:errorcluster)  [unwired: 1 in, 1 out]
        n48 = String To Path(string=w120) -> (path=w125:path)
        n49 = property on="BMSliderVert(V)" class="Slide (strict)"(error in=w102) -> (error out=w101:errorcluster, "Value"=w104:dbl)  [unwired: 1 in, 1 out]
        n50 = call <vilib>:"Open_Create_Replace File.vi"("function (open:0)"=T19."create or replace", "file path"=w125) -> ("refnum"=w117:refnum<file>)  [unwired: 6 in, 3 out]
        n51 = property on="PMHorizSlider(V)" class="Slide (strict)"(error in=w101, "Value"=w104) -> (error out=w99:errorcluster)  [unwired: 1 in, 1 out]
        n52 = property on="SampRate/Ch" class="DigNum (strict)"(error in=w99) -> (error out=w98:errorcluster, "Value"=w107:dbl)  [unwired: 1 in, 1 out]
        n53 = call-poly <vilib>:"DAQmx Timing.vi"("task/channels in"=w109, "sample mode"=w113, "samples per channel"=w108, "rate"=w107, "error in"=w98) -> ("task out"=w118:refnum<k21>, "error out"=w119:errorcluster)  [unwired: 9 in]
        n54 = call <vilib>:"DAQmx Start Task.vi"("task/channels in"=w118, "error in"=w119) -> ("task out"=w111:refnum<k21>, "error out"=w110:errorcluster)  [unwired: 12 in]
        n55 = while {
          tunnel: w110 -> [w142]
          tunnel: w111 -> [w141]
          tunnel: [w140] -> w112
          tunnel: w117 -> [w138]
          tunnel: [w137] -> w114
          tunnel: [w135] -> w116
          tunnel: w108 -> [w129]
          stop <- w127 stop-if-true
          w139 = 10.0  # Timeout
          n56 = call-poly <vilib>:"DAQmx Read.vi"("task/channels in"=w141, "number of samples per channel"=w129, "timeout"=w139, "error in"=w142) -> ("task out"=w140:refnum<k21>, "data"=w132:dbl[][], "error out"=w136:errorcluster)  [unwired: 9 in]
          n57 = for {
            N: 8 -> [_]
            tunnel: [w144] -> w133 mode=indexing
            tunnel: w132 -> [w143] mode=indexing
            n58 = call-poly <vilib>:"Mean.vi"("X"=w143) -> ("mean"=w144:dbl)  [unwired: 1 out]
          }
          n59 = To Single Precision Float(number=w133) -> (single precision float=w130:sgl[])
          n60 = call <vilib>:"Write File+ [SGL].vi"("1D array"=w130, "error in (no error)"=w136, "refnum"=w138) -> ("error out"=w135:errorcluster, "dup refnum"=w137:refnum<file>)  [unwired: 6 in, 1 out]
          n61 = Array To Cluster(array=w130) -> (cluster=→"Waveform Chart":T15)
          n62 = property on="IsPassiveModeActive?" class="Bool (strict)"() -> ("Value"=w128:bool)  [unwired: 2 in, 2 out]
          n63 = Not(x=w128) -> (.not. x?=w127:bool)
        }
        n64 = Close File(refnum=w114, error in=w116) -> (error out=w115:errorcluster)  [unwired: 1 out]
        n65 = call <vilib>:"DAQmx Stop Task.vi"("task/channels in"=w112, "error in"=w115) -> ("task out"=w106:refnum<k21>, "error out"=w92:errorcluster)  [unwired: 12 in]
        n66 = property on="PMHorizSlider(V)" class="Slide (strict)"(error in=w92) -> (error out=w95:errorcluster, "Value"=w97:dbl)  [unwired: 1 in, 1 out]
        n67 = property on="BMHorizSlider(V)" class="Slide (strict)"(error in=w95, "Value"=w97) -> (error out=w94:errorcluster)  [unwired: 1 in, 1 out]
        n68 = property on="PMVertSlider(V)" class="Slide (strict)"(error in=w94) -> (error out=w93:errorcluster, "Value"=w96:dbl)  [unwired: 1 in, 1 out]
        n69 = property on="BMSliderVert(V)" class="Slide (strict)"(error in=w93, "Value"=w96) -> (error out=w89:errorcluster)  [unwired: 1 in, 1 out]
        n70 = property on="InstrumentMode" class="Enum (strict)"(error in=w89, "Value"=w88) -> (error out=w90:errorcluster)  [unwired: 1 in, 1 out]
        n71 = property on="InterfaceSelector" class="TabCtl (strict)"(error in=w90, "Value"=T4."Basic Operation" ("InterfaceSelector")) -> (error out=w87:errorcluster)  [unwired: 1 in, 1 out]
      }
      frame "AcquireOffsetMode" {
        w162 = T1."BasicMode" ("Value")
        w165 = dbl[] []
        w172 = 10123 items=["Finite Samples"=10178, "Continuous Samples"=10123] ("sample mode")
        # "Initialize\nCluster"
        # "After you're done with the AcquireOffsetMode, go to Basic Mode"
        n72 = Bundle(w165, w165, w165, w165) -> (w166:cluster{dbl[], dbl[], dbl[], dbl[]})  [unwired: 1 in]
        n73 = call "NameFileAndFolder.vi"("ext"="*.ofs", "Head Directory"="C:\\Data" ("path")) -> ("New Filename"=w179:string, "Sub Directory"=w180:string)
        n74 = Concatenate Strings(w180, w179) -> (w176:string)
        "OffsetFilePath" <- w176
        n75 = String To Path(string=w176) -> (path=w181:path)
        n76 = call <vilib>:"Open_Create_Replace File.vi"("function (open:0)"=T19."create or replace", "file path"=w181) -> ("refnum"=w173:refnum<file>)  [unwired: 6 in, 3 out]
        n77 = call-poly <vilib>:"DAQmx Timing.vi"("task/channels in"=w157, "sample mode"=w172, "rate"="SampRate/Ch", "error in"=w170) -> ("task out"=w174:refnum<k21>, "error out"=w175:errorcluster)  [unwired: 10 in]
        n78 = call <vilib>:"DAQmx Start Task.vi"("task/channels in"=w174, "error in"=w175) -> ("task out"=w171:refnum<k21>, "error out"=w188:errorcluster)  [unwired: 12 in]
        n79 = Obtain Queue(name (unnamed)="OffsetDAQ", element data type="InitialConst", error in (no error)=w188) -> (queue out=w164:refnum<queue>, error out=w163:errorcluster)  [unwired: 2 in, 1 out]
        n80 = while {
          shift-right: [w224] -> w146
          shift-left: w163 -> [w191]
          shift-right: [w226] -> _
          shift-left: w166 -> [w225]
          tunnel: w164 -> [w192]
          i -> [w223]
          stop <- w222 stop-if-true
          # "OM stands for \"OffsetMode\""
          # "Pull in X"
          # "AI5 Mirr X axis"
          # "AI4 Mirr Y Axis"
          # "CLEAN UP MATH"
          # ">Molecule Extension>"
          # "TrapBForce"
          # "TrapAForce"
          # ">MirrorVoltage(X/Y)>"
          # "Wait for Mirror"
          # "OffsetDataLoop"
          n81 = Dequeue Element(queue=w192, error in (no error)=w191) -> (element=w206:dbl[], error out=w213:errorcluster)  [unwired: 1 in, 2 out]
          n82 = Index Array(array=w206, index=2) -> (element=w199:dbl)
          n83 = Index Array(array=w206, index=3) -> (element=w197:dbl)
          n84 = Index Array(array=w206, index=6) -> (element=w198:dbl)
          n85 = Index Array(array=w206, index=7) -> (element=w196:dbl)
          n86 = Index Array(array=w206, index=4) -> (element=w219:dbl)
          n87 = Divide(x=w199, y=w198) -> (x/y=w212:dbl)
          n88 = Divide(x=w197, y=w196) -> (x/y=w215:dbl)
          n89 = Index Array(array=w206, index=4) -> (element=w209:dbl)
          n90 = Index Array(array=w206, index=5) -> (element=w205:dbl)
          n91 = Equal To 0?(x=w223) -> (x = 0?=w210:bool)
          n92 = case shown="True" w210 {
            tunnel: w209 -> [_ w228]
            tunnel: w205 -> [_ w227]
            frame False {
            }
            frame True {
              "OM Horiz MTA Voltage" <- w228
              "OM Vert MTA Voltage" <- w227
            }
          }
          n93 = Subtract(x=w219, y="HorizMirrOffs(V)") -> (x-y=w217:dbl)
          n94 = Multiply(x="HorizMirrCalib(nm/V)", y=w217) -> (x*y=w214:dbl)
          n95 = Quotient & Remainder(x=w223, y="#PtsToWait") -> (x-y*floor(x/y)=w220:i32)  [unwired: 1 out]
          n96 = Equal To 0?(x=w220) -> (x = 0?=w211:bool)
          n97 = case shown="True" w211 {
            tunnel: w214 -> [w243 _]
            tunnel: w212 -> [w242 _]
            tunnel: w215 -> [w241 _]
            tunnel: w209 -> [w240 _]
            tunnel: [w239 w261] -> w224
            tunnel: w213 -> [w239 w262]
            tunnel: [w233 w268] -> w226
            tunnel: w225 -> [w232 w274]
            frame False {
              # ">MirrorVoltage>"
              # ">ForceTrapB Array>"
              # ">ForceTrapA Array>"
              # ">Extension Array>"
              n98 = Unbundle(w232) -> (w234:dbl[], w231:dbl[], w230:dbl[], w229:dbl[])
              n99 = Build Array (concatenate)(w234, w243) -> (w238:dbl[])
              n100 = Build Array (concatenate)(w231, w242) -> (w237:dbl[])
              n101 = Build Array (concatenate)(w230, w241) -> (w236:dbl[])
              n102 = Build Array (concatenate)(w229, w240) -> (w235:dbl[])
              n103 = Bundle(w238, w237, w236, w235) -> (w233:cluster{dbl[], dbl[], dbl[], dbl[]})  [unwired: 1 in]
            }
            frame True {
              w269 = dbl[] []
              w246 = 1000 ("chart length (points)")
              # "Update Plots"
              n104 = Unbundle(w274) -> (w273:dbl[], w272:dbl[], w271:dbl[], w270:dbl[])
              n105 = call-poly <vilib>:"Mean.vi"("X"=w270) -> ()  [unwired: 2 out]
              n106 = call <vilib>:"Std Deviation and Variance.vi"("X"=w273) -> ("mean"=w275:dbl, "standard deviation"=w276:dbl)  [unwired: 1 in, 1 out]
              n107 = call-poly <vilib>:"Mean.vi"("X"=w271) -> ("mean"=w281:dbl)  [unwired: 1 out]
              n108 = call-poly <vilib>:"DAQmx Create Virtual Channel.vi"("maximum value"=10.0 ("Maximum Value"), "minimum value"=0.0 ("Minimum Value"), "physical channels"=tag "PCI-6036E/ao0", "error in"=w262) -> ("task out"=w254:refnum<k21>, "error out"=w253:errorcluster)  [unwired: 10 in]
              n109 = property on="OM Horiz MTA Voltage" class="DigNum (strict)"() -> ("Value"=w258:dbl)  [unwired: 2 in, 2 out]
              n110 = call-poly <vilib>:"Mean.vi"("X"=w272) -> ("mean"=w280:dbl)  [unwired: 1 out]
              n111 = Bundle("mean"=w275, "standard deviation"=w276) -> (w251:cluster{"mean":dbl, "standard deviation":dbl})  [unwired: 1 in]
              n112 = Bundle("mean"=w275, "mean"=w280) -> (w250:cluster{"mean":dbl, "mean":dbl})  [unwired: 1 in]
              n113 = Bundle("mean"=w275, "mean"=w281) -> (w248:cluster{"mean":dbl, "mean":dbl})  [unwired: 1 in]
              n114 = Build Array(w250) -> (w249:cluster{"mean":dbl, "mean":dbl}[])
              n115 = Build Array(w251) -> (w245:cluster{"mean":dbl, "standard deviation":dbl}[])
              n116 = Build Array(w248) -> (w247:cluster{"mean":dbl, "mean":dbl}[])
              n117 = Subtract(x=w258, y="Step (V)") -> (x-y=w279:dbl)
              n118 = In Range and Coerce(upper limit=10.0, x=w279, lower limit=0.0 ("upper limit")) -> (coerced(x)=w260:dbl)  [unwired: 1 out]
              n119 = call <instrlib>:"XY Chart Buffer.vi"("Clear First?"="ClearChart", "Chart Length"=w246, "New Points"=w245) -> ("XY Chart Data"=→"Noise-Ext":cluster{"x":dbl[], "y":dbl[]}[])  [unwired: 7 in, 1 out]
              n120 = call <instrlib>:"XY Chart Buffer.vi"("Clear First?"="ClearChart", "Chart Length"=w246, "New Points"=w249) -> ("XY Chart Data"=→"Force TrapA":cluster{"x":dbl[], "y":dbl[]}[])  [unwired: 7 in, 1 out]
              n121 = call <instrlib>:"XY Chart Buffer.vi"("Clear First?"="ClearChart", "Chart Length"=w246, "New Points"=w247) -> ("XY Chart Data"=→"Force TrapB":cluster{"x":dbl[], "y":dbl[]}[])  [unwired: 7 in, 1 out]
              n122 = call-poly <vilib>:"DAQmx Write.vi"("task/channels in"=w254, "data"=w260, "timeout"=10.0, "error in"=w253) -> ("task out"=w266:refnum<k21>, "error out"=w267:errorcluster)  [unwired: 9 in, 1 out]
              n123 = property on="OM Horiz MTA Voltage" class="DigNum (strict)"("Value"=w260) -> ()  [unwired: 2 in, 2 out]
              n124 = call <vilib>:"DAQmx Clear Task.vi"("task in"=w266, "error in"=w267) -> ("error out"=w261:errorcluster)  [unwired: 13 in]
              n125 = Bundle(w269, w269, w269, w269) -> (w268:cluster{dbl[], dbl[], dbl[], dbl[]})  [unwired: 1 in]
            }
          }
          n126 = property on="OM Horiz MTA Voltage" class="DigNum (strict)"() -> ("Value"=w193:dbl)  [unwired: 2 in, 2 out]
          n127 = Less Or Equal?(x=w193, y="Stop Voltage (V)") -> (x <= y?=w195:bool)
          n128 = property on="IsOffsetModeActive?" class="Bool (strict)"() -> ("Value"=w190:bool)  [unwired: 2 in, 2 out]
          n129 = Not(x=w190) -> (.not. x?=w189:bool)
          n130 = Compound Arithmetic op=OR(w189, w195) -> (w222:bool)
        }
        n131 = while {
          tunnel: w171 -> [w303]
          tunnel: [w302] -> w169
          tunnel: w173 -> [w293]
          tunnel: "AveragingWindow" -> [w298]
          tunnel: w164 -> [w297]
          shift-right: [w289] -> w168
          shift-left: w163 -> [w304]
          tunnel: [w295] -> w187
          tunnel: [w288] -> w167
          stop <- w284 stop-if-true
          w301 = 10.0  # Timeout
          # "Enque Data"
          n132 = call-poly <vilib>:"DAQmx Read.vi"("task/channels in"=w303, "number of samples per channel"=w298, "timeout"=w301, "error in"=w304) -> ("task out"=w302:refnum<k21>, "data"=w299:dbl[][], "error out"=w291:errorcluster)  [unwired: 9 in]
          n133 = for {
            N: 8 -> [_]
            tunnel: [w306] -> w294 mode=indexing
            tunnel: w299 -> [w305] mode=indexing
            n134 = call-poly <vilib>:"Mean.vi"("X"=w305) -> ("mean"=w306:dbl)  [unwired: 1 out]
          }
          n135 = To Single Precision Float(number=w294) -> (single precision float=w292:sgl[])
          n136 = Write to Binary File(file (use dialog)=w293, data=w292, error in=w291) -> (refnum out=w288:refnum<file>, error out=w290:errorcluster)  [unwired: 3 in, 1 out]
          n137 = Enqueue Element(queue=w297, element=w294, error in (no error)=w291) -> (queue out=w295:refnum<queue>, error out=w296:errorcluster)  [unwired: 1 in, 1 out]
          n138 = Merge Errors(w290, w296) -> (w289:errorcluster)
          n139 = property on="IsOffsetModeActive?" class="Bool (strict)"() -> ("Value"=w283:bool)  [unwired: 2 in, 2 out]
          n140 = property on="OM Horiz MTA Voltage" class="DigNum (strict)"() -> ("Value"=w286:dbl)  [unwired: 2 in, 2 out]
          n141 = property on="Stop Voltage (V)" class="DigNum (strict)"() -> ("Value"=w287:dbl)  [unwired: 2 in, 2 out]
          n142 = Not(x=w283) -> (.not. x?=w282:bool)
          n143 = Less Or Equal?(x=w286, y=w287) -> (x <= y?=w285:bool)
          n144 = Compound Arithmetic op=OR(w282, w285) -> (w284:bool)
        }
        n145 = call <vilib>:"DAQmx Stop Task.vi"("task/channels in"=w169, "error in"=w168) -> ("task out"=w152:refnum<k21>, "error out"=w151:errorcluster)  [unwired: 12 in]
        n146 = Close File(refnum=w167) -> (error out=w156:errorcluster)  [unwired: 1 in, 1 out]
        n147 = Release Queue(queue=w187, error in (no error)=w151) -> (error out=w148:errorcluster)  [unwired: 1 in, 2 out]
        n148 = property on="InstrumentMode" class="Enum (strict)"(error in=w156, "Value"=w162) -> (error out=w160:errorcluster)  [unwired: 1 in, 1 out]
        n149 = property on="SampRate/Ch" class="DigNum (strict)"() -> ("Value"=w153:dbl)  [unwired: 2 in, 2 out]
        n150 = call "GetTrapSeparation(V).vi"("ErrorIn"=w148, "AcquisitionRatePerChannel"=w153, "DAQ Task"=w152) -> ("ErrorOut"=w149:errorcluster, "VertTrapSeparation(V)"=w155:dbl, "HorTrapSeparation(V)"=w154:dbl, "DAQ Task"=w150:refnum<k21>)  [unwired: 1 in]
        n151 = property on="InterfaceSelector" class="TabCtl (strict)"(error in=w160, "Value"=T4."Basic Operation" ("InterfaceSelector")) -> (error out=w158:errorcluster)  [unwired: 1 in, 1 out]
        n152 = property on="BMSliderVert(V)" class="Slide (strict)"("Value"=w155) -> ()  [unwired: 2 in, 2 out]
        n153 = property on="BMHorizSlider(V)" class="Slide (strict)"("Value"=w154) -> ()  [unwired: 2 in, 2 out]
        n154 = property on="IsOffsetModeActive?" class="Bool (strict)"(error in=w158, "Value"=FALSE ("IsOffsetModeActive?")) -> (error out=w147:errorcluster)  [unwired: 1 in, 1 out]
        n155 = Merge Errors(w147, w149, w146) -> (w145:errorcluster)
      }
      frame "AcquireSpectrumMode" {
        w320 = T1."BasicMode"
        w329 = 10123 items=["Finite Samples"=10178, "Continuous Samples"=10123] ("sample mode")
        # "Gheorghe Chistol\n090512"
        n156 = call-poly <vilib>:"DAQmx Timing.vi"("task/channels in"=w308, "sample mode"=w329, "samples per channel"="WindowSample#", "rate"="HiFSamplingRate/Ch", "error in"=w327) -> ("task out"=w312:refnum<k21>, "error out"=w311:errorcluster)  [unwired: 9 in]
        n157 = call <vilib>:"DAQmx Start Task.vi"("task/channels in"=w312, "error in"=w311) -> ("task out"=w310:refnum<k21>, "error out"=w313:errorcluster)  [unwired: 12 in]
        n158 = property on="HiFreqDiagnostic" class="WFChart (strict)"("XScale.Maximum"="Total#OfWindows") -> (error out=w342:errorcluster)  [unwired: 2 in, 1 out]
        n159 = property on="ProgressBar" class="Slide (strict)"(error in=w313, "Scale.Maximum"="Total#OfWindows") -> (error out=w339:errorcluster)  [unwired: 1 in, 1 out]
        n160 = call "NameFileAndFolder.vi"("ext"="*.brw", "Head Directory"="C:\\Data" ("path")) -> ("New Filename"=w333:string, "Sub Directory"=w334:string)
        n161 = Concatenate Strings(w334, w333) -> (w330:string)
        "File Name and Path" <- w330
        n162 = property on="HiFreqDiagnostic" class="WFChart (strict)"(error in=w342, "XScale.Minimum"=0.0 ("X Scale.Range:Minimum")) -> (error out=w345:errorcluster)  [unwired: 1 in, 1 out]
        n163 = property on="ProgressBar" class="Slide (strict)"(error in=w339, "Scale.Minimum"=0.0 ("Scale.Range:Minimum")) -> (error out=w317:errorcluster)  [unwired: 1 in, 1 out]
        n164 = String To Path(string=w330) -> (path=w335:path)
        n165 = call <vilib>:"Open_Create_Replace File.vi"("error in (no error)"=w317, "function (open:0)"=T19."create or replace", "file path"=w335) -> ("error out"=w316:errorcluster, "refnum"=w338:refnum<file>)  [unwired: 5 in, 2 out]
        n166 = property on="HiFreqDiagnostic" class="WFChart (strict)"(error in=w345, "History Data"=T20 []) -> ()  [unwired: 1 in, 2 out]
        n167 = while {
          tunnel: [w364] -> w328
          tunnel: w310 -> [w361]
          tunnel: w338 -> [w358]
          tunnel: "Total#OfWindows" -> [w357]
          shift-right: [w359] -> w315
          shift-left: w316 -> [w360]
          tunnel: "WindowSample#" -> [w347]
          tunnel: [w346] -> w314
          i -> [w354]
          stop <- w348 stop-if-true
          # "Saving in Single Saves Space on Disk"
          n168 = To Long Integer(number=w357) -> (32bit integer=w355:i32)
          n169 = call-poly <vilib>:"DAQmx Read.vi"("task/channels in"=w361, "number of samples per channel"=w347, "timeout"=10.0, "error in"=w360) -> ("task out"=w346:refnum<k21>, "data"=w351:dbl[][], "error out"=w363:errorcluster)  [unwired: 9 in]
          n170 = Equal?(x=w355, y=w354) -> (x = y?=w348:bool)
          n171 = Transpose 2D Array(2D array=w351) -> (transposed array=w350:dbl[][])
          n172 = To Single Precision Float(number=w350) -> (single precision float=w349:sgl[][])
          n173 = for {
            N: 8 -> [_]
            tunnel: [w367] -> w353 mode=indexing
            tunnel: w351 -> [w366] mode=indexing
            n174 = call-poly <vilib>:"Mean.vi"("X"=w366) -> ("mean"=w367:dbl)  [unwired: 1 out]
          }
          n175 = Write to Binary File(file (use dialog)=w358, data=w349, error in=w363, 5:FALSE ("prepend array or string size? (T)")) -> (refnum out=w364:refnum<file>, error out=w359:errorcluster)  [unwired: 2 in, 1 out]
          n176 = Array To Cluster(array=w353) -> (cluster=→"HiFreqDiagnostic":T16)
          "ProgressBar" <- w354
        }
        n177 = call <vilib>:"DAQmx Stop Task.vi"("task/channels in"=w314, "error in"=w315) -> ("task out"=w307:refnum<k21>, "error out"=w309:errorcluster)  [unwired: 12 in]
        n178 = Close File(refnum=w328, error in=w309) -> (error out=w326:errorcluster)  [unwired: 1 out]
        n179 = property on="InstrumentMode" class="Enum (strict)"(error in=w326, "Value"=w320) -> (error out=w324:errorcluster)  [unwired: 1 in, 1 out]
        n180 = property on="InterfaceSelector" class="TabCtl (strict)"(error in=w324, "Value"=T4."Basic Operation" ("InterfaceSelector")) -> (error out=w322:errorcluster)  [unwired: 1 in, 1 out]
        n181 = Unbundle By Name(w322) -> ("status"=w321:bool)
        n182 = Select(t=T1."Shutdown", s=w321, f=w320) -> (s? t:f=w318:T1)
      }
      frame "Force-ExtensionMode" {
        w379 = T1."BasicMode" ("InstrumentMode")
        w410 = dbl[] []
        w393 = 10123 items=["Finite Samples"=10178, "Continuous Samples"=10123] ("sample mode")
        # "Initialize\nCluster"
        n183 = property on="SampRate/Ch" class="DigNum (strict)"() -> ("Value"=w391:dbl)  [unwired: 2 in, 2 out]
        n184 = property on="AveragingWindow" class="DigNum (strict)"() -> ("Value"=w368:i32)  [unwired: 2 in, 2 out]
        n185 = call-poly <vilib>:"DAQmx Timing.vi"("task/channels in"=w382, "sample mode"=w393, "samples per channel"=w368, "rate"=w391, "error in"=w390) -> ("task out"=w396:refnum<k21>, "error out"=w397:errorcluster)  [unwired: 9 in]
        n186 = call "NameFileAndFolder.vi"("ext"="*.pulling", "Head Directory"="C:\\Data" ("path")) -> ("New Filename"=w401:string, "Sub Directory"=w402:string)
        n187 = call <vilib>:"DAQmx Start Task.vi"("task/channels in"=w396, "error in"=w397) -> ("task out"=w392:refnum<k21>, "error out"=w407:errorcluster)  [unwired: 12 in]
        n188 = Concatenate Strings(w402, w401) -> (w398:string)
        "ForceExtensionFilePath" <- w398
        n189 = Obtain Queue(name (unnamed)="ForceExtDAQ", element data type="ForceExtInitConst", error in (no error)=w407) -> (queue out=w409:refnum<queue>, error out=w389:errorcluster)  [unwired: 2 in, 1 out]
        n190 = Bundle(w410, w410, w410, w410) -> (w411:cluster{dbl[], dbl[], dbl[], dbl[]})  [unwired: 1 in]
        n191 = String To Path(string=w398) -> (path=w403:path)
        n192 = while {
          shift-right: [w453] -> w370
          shift-left: w389 -> [w435]
          tunnel: w409 -> [w460]
          shift-right: [w456] -> _
          shift-left: w411 -> [w455]
          i -> [w451]
          stop <- w433 stop-if-true
          # "Pull in X"
          # "AI5 Mirr X axis\n(vertical trap motion)"
          # "AI4 Mirr Y Axis\n(horizontal trap motion)"
          # "Finish The Math Here"
          # ">Molecule Extension>"
          # "TrapBForce"
          # "TrapAForce"
          # ">MirrorVoltage(X/Y)>"
          # "Wait for Mirror"
          n193 = Dequeue Element(queue=w460, error in (no error)=w435) -> (element=w446:dbl[], error out=w457:errorcluster)  [unwired: 1 in, 2 out]
          n194 = Index Array(array=w446, index=2) -> (element=w439:dbl)
          n195 = Index Array(array=w446, index=3) -> (element=w437:dbl)
          n196 = Index Array(array=w446, index=6) -> (element=w438:dbl)
          n197 = Index Array(array=w446, index=7) -> (element=w436:dbl)
          n198 = Index Array(array=w446, index=4) -> (element=w464:dbl)
          n199 = Divide(x=w439, y=w438) -> (x/y=w454:dbl)
          n200 = Divide(x=w437, y=w436) -> (x/y=w459:dbl)
          n201 = Index Array(array=w446, index=4) -> (element=w449:dbl)
          n202 = Index Array(array=w446, index=5) -> (element=w445:dbl)
          n203 = Equal To 0?(x=w451) -> (x = 0?=w450:bool)
          n204 = case shown="True" w450 {
            tunnel: w449 -> [_ w468]
            tunnel: w445 -> [_ w467]
            frame False {
            }
            frame True {
              "FEX Mirror Y Volt" <- w468
              "FEX Mirror X Volt" <- w467
            }
          }
          n205 = Subtract(x=w464, y="FEX HorizMirrOffs(V)") -> (x-y=w462:dbl)
          n206 = Multiply(x="FEX HorizMirrCalib(nm/V)", y=w462) -> (x*y=w458:dbl)
          n207 = Quotient & Remainder(x=w451, y="#FEXPtsToWait") -> (x-y*floor(x/y)=w465:i32)  [unwired: 1 out]
          n208 = Equal To 0?(x=w465) -> (x = 0?=w452:bool)
          n209 = case shown="True" w452 {
            tunnel: w458 -> [w483 _]
            tunnel: w454 -> [w482 _]
            tunnel: w459 -> [w481 _]
            tunnel: w449 -> [w480 _]
            tunnel: [w479 w491] -> w453
            tunnel: w457 -> [w479 w492]
            tunnel: [w473 w498] -> w456
            tunnel: w455 -> [w472 w504]
            frame False {
              # ">MirrorVoltage>"
              # ">ForceTrapB Array>"
              # ">ForceTrapA Array>"
              # ">Extension Array>"
              n210 = Unbundle(w472) -> (w474:dbl[], w471:dbl[], w470:dbl[], w469:dbl[])
              n211 = Build Array (concatenate)(w474, w483) -> (w478:dbl[])
              n212 = Build Array (concatenate)(w471, w482) -> (w477:dbl[])
              n213 = Build Array (concatenate)(w470, w481) -> (w476:dbl[])
              n214 = Build Array (concatenate)(w469, w480) -> (w475:dbl[])
              n215 = Bundle(w478, w477, w476, w475) -> (w473:cluster{dbl[], dbl[], dbl[], dbl[]})  [unwired: 1 in]
            }
            frame True {
              w499 = dbl[] []
              (unwired) 1000 ("chart length (points)")
              n216 = Unbundle(w504) -> (w503:dbl[], w502:dbl[], w501:dbl[], w500:dbl[])
              n217 = call-poly <vilib>:"Mean.vi"("X"=w500) -> ()  [unwired: 2 out]
              n218 = Select(t=1.0, s="Direction", f=-1.0) -> (s? t:f=w505:dbl)
              n219 = call <vilib>:"Std Deviation and Variance.vi"("X"=w503) -> ("mean"=w513:dbl, "standard deviation"=w517:dbl)  [unwired: 1 in, 1 out]
              n220 = call-poly <vilib>:"Mean.vi"("X"=w501) -> ("mean"=w522:dbl)  [unwired: 1 out]
              n221 = Select(t=1.0, s="IsPullActive?", f=0.0) -> (s? t:f=w506:dbl)
              n222 = call-poly <vilib>:"Mean.vi"("X"=w502) -> ("mean"=w521:dbl)  [unwired: 1 out]
              n223 = Multiply(x=w506, y=w505) -> (x*y=w515:dbl)
              n224 = property on="FEX Mirror Y Volt" class="DigNum (strict)"() -> ("Value"=w487:dbl)  [unwired: 2 in, 2 out]
              n225 = call-poly <vilib>:"DAQmx Create Virtual Channel.vi"("maximum value"=10.0 ("Maximum Value"), "minimum value"=0.0 ("Minimum Value"), "physical channels"=tag "PCI-6036E/ao0", "error in"=w492) -> ("task out"=w485:refnum<k21>, "error out"=w484:errorcluster)  [unwired: 10 in]
              n226 = Bundle("mean"=w513, "standard deviation"=w517) -> ()  [unwired: 1 in, 1 out]
              n227 = Bundle("mean"=w513, "mean"=w521) -> ()  [unwired: 1 in, 1 out]
              n228 = Bundle("mean"=w513, "mean"=w522) -> ()  [unwired: 1 in, 1 out]
              n229 = Multiply(x="Mirror Step (V)", y=w515) -> (x*y=w514:dbl)
              n230 = call <instrlib>:"XY Chart Buffer.vi"() -> ("XY Chart Data"=→"FEX Noise-Ext":cluster{"x":dbl[], "y":dbl[]}[])  [unwired: 10 in, 1 out]
              n231 = call <instrlib>:"XY Chart Buffer.vi"() -> ("XY Chart Data"=→"FEX Force TrapA":cluster{"x":dbl[], "y":dbl[]}[])  [unwired: 10 in, 1 out]
              n232 = Add(x=w487, y=w514) -> (x+y=w520:dbl)
              n233 = In Range and Coerce(upper limit=10.0, x=w520, lower limit=0.0 ("upper limit")) -> (coerced(x)=w490:dbl)  [unwired: 1 out]
              n234 = call-poly <vilib>:"DAQmx Write.vi"("task/channels in"=w485, "data"=w490, "timeout"=10.0, "error in"=w484) -> ("task out"=w496:refnum<k21>, "error out"=w497:errorcluster)  [unwired: 9 in, 1 out]
              n235 = property on="FEX MirrorY Volt" class="DigNum (strict)"("Value"=w490) -> ()  [unwired: 2 in, 2 out]
              n236 = call <vilib>:"DAQmx Clear Task.vi"("task in"=w496, "error in"=w497) -> ("error out"=w491:errorcluster)  [unwired: 13 in]
              n237 = Bundle(w499, w499, w499, w499) -> (w498:cluster{dbl[], dbl[], dbl[], dbl[]})  [unwired: 1 in]
            }
          }
          n238 = property on="IsForceExtActive?" class="Bool (strict)"() -> ("Value"=w434:bool)  [unwired: 2 in, 2 out]
          n239 = Not(x=w434) -> (.not. x?=w433:bool)
        }
        n240 = call <vilib>:"Open_Create_Replace File.vi"("function (open:0)"=T19."create or replace", "file path"=w403) -> ("refnum"=w395:refnum<file>)  [unwired: 6 in, 3 out]
        n241 = while {
          tunnel: w392 -> [w429]
          tunnel: [w428] -> w384
          tunnel: w395 -> [w426]
          tunnel: [w425] -> w394
          tunnel: w368 -> [w422]
          tunnel: w409 -> [w421]
          shift-right: [w417] -> w381
          shift-left: w389 -> [w430]
          tunnel: [w416] -> w408
          stop <- w412 stop-if-true
          w427 = 10.0  # Timeout
          # "Enque Data"
          # "Force-Extension DAQ Loop"
          n242 = call-poly <vilib>:"DAQmx Read.vi"("task/channels in"=w429, "number of samples per channel"=w422, "timeout"=w427, "error in"=w430) -> ("task out"=w428:refnum<k21>, "data"=w423:dbl[][], "error out"=w420:errorcluster)  [unwired: 9 in]
          n243 = for {
            N: 8 -> [_]
            tunnel: [w432] -> w414 mode=indexing
            tunnel: w423 -> [w431] mode=indexing
            n244 = call-poly <vilib>:"Mean.vi"("X"=w431) -> ("mean"=w432:dbl)  [unwired: 1 out]
          }
          n245 = To Single Precision Float(number=w414) -> (single precision float=w415:sgl[])
          n246 = call <vilib>:"Write File+ [SGL].vi"("1D array"=w415, "error in (no error)"=w420, "refnum"=w426) -> ("error out"=w419:errorcluster, "dup refnum"=w425:refnum<file>)  [unwired: 6 in, 1 out]
          n247 = Enqueue Element(queue=w421, element=w414, error in (no error)=w420) -> (queue out=w416:refnum<queue>, error out=w418:errorcluster)  [unwired: 1 in, 1 out]
          n248 = property on="IsForceExtActive?" class="Bool (strict)"() -> ("Value"=w413:bool)  [unwired: 2 in, 2 out]
          n249 = Not(x=w413) -> (.not. x?=w412:bool)
          n250 = Merge Errors(w419, w418) -> (w417:errorcluster)
        }
        n251 = call <vilib>:"DAQmx Stop Task.vi"("task/channels in"=w384, "error in"=w381) -> ("task out"=w375:refnum<k21>, "error out"=w383:errorcluster)  [unwired: 12 in]
        n252 = Close File(refnum=w394) -> (error out=w380:errorcluster)  [unwired: 1 in, 1 out]
        n253 = Release Queue(queue=w408, error in (no error)=w383) -> (error out=w374:errorcluster)  [unwired: 1 in, 2 out]
        n254 = property on="InstrumentMode" class="Enum (strict)"(error in=w380, "Value"=w379) -> (error out=w388:errorcluster)  [unwired: 1 in, 1 out]
        n255 = property on="InterfaceSelector" class="TabCtl (strict)"(error in=w388, "Value"=T4."Basic Operation" ("InterfaceSelector")) -> (error out=w387:errorcluster)  [unwired: 1 in, 1 out]
        n256 = property on="IsForceExtActive?" class="Bool (strict)"(error in=w387, "Value"=FALSE ("IsOffsetModeActive?")) -> (error out=w371:errorcluster)  [unwired: 1 in, 1 out]
        n257 = property on="SampRate/Ch" class="DigNum (strict)"() -> ("Value"=w378:dbl)  [unwired: 2 in, 2 out]
        n258 = call "GetTrapSeparation(V).vi"("ErrorIn"=w374, "AcquisitionRatePerChannel"=w378, "DAQ Task"=w375) -> ("ErrorOut"=w372:errorcluster, "VertTrapSeparation(V)"=w376:dbl, "HorTrapSeparation(V)"=w377:dbl, "DAQ Task"=w373:refnum<k21>)  [unwired: 1 in]
        n259 = property on="BMSliderVert(V)" class="Slide (strict)"("Value"=w376) -> ()  [unwired: 2 in, 2 out]
        n260 = property on="BMHorizSlider(V)" class="Slide (strict)"("Value"=w377) -> ()  [unwired: 2 in, 2 out]
        n261 = Merge Errors(w371, w372, w370) -> (w369:errorcluster)
      }
      frame "Shutdown" {
        n262 = Wait (ms)(milliseconds to wait=u32 25) -> ()  [unwired: 1 out]
        n263 = call <vilib>:"DAQmx Clear Task.vi"("task in"=w523, "error in"=w526) -> ("error out"=w525:errorcluster)  [unwired: 13 in]
        n264 = property on="InstrumentMode" class="Enum (strict)"(error in=w525) -> (error out=w524:errorcluster, "Value"=w528:T1)  [unwired: 1 in, 1 out]
      }
    }
  }
  n265 = while {
    shift-right: [w535] -> w1
    shift-left: _ -> [w534]
    tunnel: w9 -> [w533]
    i -> [w531]
    stop <- w532 stop-if-true
    # "UI Loop"
    n266 = Wait (ms)(milliseconds to wait=u32 10) -> ()  [unwired: 1 out]
    n267 = event shown="[4] \"GoToTopDisp\": Value Change" {
      selector: _ -> [_ _ _ _ _ _ _ _ _ _ _ _ _ _ _ _]
      dyn-events: _ -> [_ _ _ _ _ _ _ _ _ _ _ _ _ _ _ _]
      timeout: 10 -> [_ _ _ _ _ _ _ _ _ _ _ _ _ _ _ _]
      tunnel: [_ w567 w596 w625 w664 w730 w796 w850 w860 w870 _ _ _ _ _ w922] -> w535
      tunnel: w534 -> [_ w566 w595 w624 w663 w729 w795 w853 w863 w870 _ _ _ _ _ w922]
      tunnel: [_ _ _ _ _ _ _ _ _ _ _ _ _ _ _ "Stop"] -> w532
      tunnel: w533 -> [_ w565 w594 w623 w662 w728 w794 _ _ _ _ _ _ _ _ _]
      tunnel: w531 -> [w538 _ _ _ _ _ _ _ _ _ _ _ _ _ _ _]
      event Timeout {
        n268 = event-data() -> ()  [unwired: 1 in, 1 out]
        n269 = case shown="True" "Oscillate Mirror?" {
          selector: "Oscillate Mirror?" -> [_ w553]
          tunnel: w538 -> [_ w554]
          frame False {
          }
          frame True {
            w563 = 100
            # "Enforce Upper/Lower Bounds"
            n270 = Multiply(x="Period (s)", y=1000) -> (x*y=w561:i32)
            n271 = Divide(x=6.283185307179586, y=w563) -> (x/y=w557:dbl)
            n272 = Divide(x=w561, y=w563) -> (x/y=w562:dbl)
            n273 = Multiply(x=w557, y=w554) -> (x*y=w558:dbl)
            n274 = Wait (ms)(milliseconds to wait=w562) -> ()  [unwired: 1 out]
            n275 = Sine(x=w558) -> (sin(x)=w559:dbl)
            n276 = Multiply(x="Amplitude (V)", y=w559) -> (x*y=w551:dbl)
            n277 = Add(x=w551, y="Offset (V)") -> (x+y=w539:dbl)
            "Mirror Voltage" <- w539
            n278 = property on="BMHorizSlider(V)" class="Slide (strict)"("Value"=w539) -> ()  [unwired: 2 in, 2 out]
            n279 = call-poly <vilib>:"DAQmx Create Virtual Channel.vi"("maximum value"=10.0 ("Maximum Value"), "minimum value"=0.0 ("Minimum Value"), "physical channels"=tag "PCI-6036E/ao0") -> ("task out"=w541:refnum<k21>, "error out"=w540:errorcluster)  [unwired: 11 in]
            n280 = In Range and Coerce(upper limit=10.0, x=w539, lower limit=0.0 ("upper limit")) -> (coerced(x)=w545:dbl)  [unwired: 1 out]
            n281 = call-poly <vilib>:"DAQmx Write.vi"("task/channels in"=w541, "data"=w545, "timeout"=10.0, "error in"=w540) -> ("task out"=w543:refnum<k21>, "error out"=w542:errorcluster)  [unwired: 9 in, 1 out]
            n282 = call <vilib>:"DAQmx Clear Task.vi"("task in"=w543, "error in"=w542) -> ()  [unwired: 13 in, 1 out]
            "Oscillate Mirror? 2" <- w553
          }
        }
      }
      event "SaveTopDisp": Value Change {
        n283 = event-data() -> ()  [unwired: 1 in, 1 out]
        n284 = property on="IsActive?" class="Bool (strict)"(error in=w566) -> (error out=w574:errorcluster, "Value"=w572:bool)  [unwired: 1 in, 1 out]
        n285 = property on="IsActive?" class="Bool (strict)"(error in=w574) -> (error out=w573:errorcluster, "Value"=w571:bool)  [unwired: 1 in, 1 out]
        n286 = property on="IsActive?" class="Bool (strict)"(error in=w573) -> (error out=w568:errorcluster, "Value"=w570:bool)  [unwired: 1 in, 1 out]
        n287 = Compound Arithmetic op=AND(w572, w571, w570) -> (w569:bool)
        n288 = case shown="True" w569 {
          tunnel: w568 -> [w575 w593]
          tunnel: [w575 w580] -> w567
          tunnel: w565 -> [_ w579]
          frame False {
          }
          frame True {
            # "Read the Current Motor Positions and save them to the Top Dispenser"
            # "X Motor Pos"
            # "Y Motor Pos"
            # "Z Motor Pos"
            n289 = Unbundle(w579) -> ("XMotorRef"=w576:refnum<k7>, "YMotorRef"=w577:refnum<k7>, "ZMotorRef"=w578:refnum<k7>)
            n290 = invoke class="MG17Motor" method="GetPosition_Position"(reference=w578, error in=w593, "lChanID"=0) -> (error out=w590:errorcluster, "GetPosition_Position"=w583:sgl)  [unwired: 1 in, 2 out]
            n291 = invoke class="MG17Motor" method="GetPosition_Position"(reference=w577, error in=w590, "lChanID"=0) -> (error out=w588:errorcluster, "GetPosition_Position"=w582:sgl)  [unwired: 1 in, 2 out]
            n292 = invoke class="MG17Motor" method="GetPosition_Position"(reference=w576, error in=w588, "lChanID"=0) -> (error out=w587:errorcluster, "GetPosition_Position"=w581:sgl)  [unwired: 1 in, 2 out]
            n293 = property on="Top Dispenser" class="Clust (strict)"(error in=w587) -> (error out=w586:errorcluster, "Value"=w585:T5)  [unwired: 1 in, 1 out]
            n294 = Bundle By Name(cluster=w585, "X Pos (mm)"=w581, "Y Pos (mm)"=w582, "Z Pos (mm)"=w583) -> (w584:T5)
            n295 = property on="Top Dispenser" class="Clust (strict)"(error in=w586, "Value"=w584) -> (error out=w580:errorcluster)  [unwired: 1 in, 1 out]
          }
        }
      }
      event "SaveBottDisp": Value Change {
        n296 = event-data() -> ()  [unwired: 1 in, 1 out]
        n297 = property on="IsActive?" class="Bool (strict)"(error in=w595) -> (error out=w603:errorcluster, "Value"=w601:bool)  [unwired: 1 in, 1 out]
        n298 = property on="IsActive?" class="Bool (strict)"(error in=w603) -> (error out=w602:errorcluster, "Value"=w600:bool)  [unwired: 1 in, 1 out]
        n299 = property on="IsActive?" class="Bool (strict)"(error in=w602) -> (error out=w597:errorcluster, "Value"=w599:bool)  [unwired: 1 in, 1 out]
        n300 = Compound Arithmetic op=AND(w601, w600, w599) -> (w598:bool)
        n301 = case shown="True" w598 {
          tunnel: w597 -> [w604 w622]
          tunnel: [w604 w609] -> w596
          tunnel: w594 -> [_ w608]
          frame False {
          }
          frame True {
            # "Read the Current Motor Positions and save them to the Bottom Dispenser"
            # "X Motor Pos"
            # "Y Motor Pos"
            # "Z Motor Pos"
            n302 = Unbundle(w608) -> ("XMotorRef"=w605:refnum<k7>, "YMotorRef"=w606:refnum<k7>, "ZMotorRef"=w607:refnum<k7>)
            n303 = invoke class="MG17Motor" method="GetPosition_Position"(reference=w607, error in=w622, "lChanID"=0) -> (error out=w619:errorcluster, "GetPosition_Position"=w612:sgl)  [unwired: 1 in, 2 out]
            n304 = invoke class="MG17Motor" method="GetPosition_Position"(reference=w606, error in=w619, "lChanID"=0) -> (error out=w617:errorcluster, "GetPosition_Position"=w611:sgl)  [unwired: 1 in, 2 out]
            n305 = invoke class="MG17Motor" method="GetPosition_Position"(reference=w605, error in=w617, "lChanID"=0) -> (error out=w616:errorcluster, "GetPosition_Position"=w610:sgl)  [unwired: 1 in, 2 out]
            n306 = property on="Bottom Dispenser" class="Clust (strict)"(error in=w616) -> (error out=w615:errorcluster, "Value"=w614:T5)  [unwired: 1 in, 1 out]
            n307 = Bundle By Name(cluster=w614, "X Pos (mm)"=w610, "Y Pos (mm)"=w611, "Z Pos (mm)"=w612) -> (w613:T5)
            n308 = property on="Bottom Dispenser" class="Clust (strict)"(error in=w615, "Value"=w613) -> (error out=w609:errorcluster)  [unwired: 1 in, 1 out]
          }
        }
      }
      event "SaveExpLoc": Value Change {
        n309 = event-data() -> ()  [unwired: 1 in, 1 out]
        n310 = property on="IsActive?" class="Bool (strict)"(error in=w624) -> (error out=w632:errorcluster, "Value"=w630:bool)  [unwired: 1 in, 1 out]
        n311 = property on="IsActive?" class="Bool (strict)"(error in=w632) -> (error out=w631:errorcluster, "Value"=w629:bool)  [unwired: 1 in, 1 out]
        n312 = property on="IsActive?" class="Bool (strict)"(error in=w631) -> (error out=w626:errorcluster, "Value"=w628:bool)  [unwired: 1 in, 1 out]
        n313 = Compound Arithmetic op=AND(w630, w629, w628) -> (w627:bool)
        n314 = case shown="True" w627 {
          tunnel: w626 -> [w633 w651]
          tunnel: [w633 w638] -> w625
          tunnel: w623 -> [_ w637]
          frame False {
          }
          frame True {
            # "Read the Current Motor Positions and save them to the Exp Location"
            # "X Motor Pos"
            # "Y Motor Pos"
            # "Z Motor Pos"
            n315 = Unbundle(w637) -> ("XMotorRef"=w634:refnum<k7>, "YMotorRef"=w635:refnum<k7>, "ZMotorRef"=w636:refnum<k7>)
            n316 = invoke class="MG17Motor" method="GetPosition_Position"(reference=w636, error in=w651, "lChanID"=0) -> (error out=w648:errorcluster, "GetPosition_Position"=w641:sgl)  [unwired: 1 in, 2 out]
            n317 = invoke class="MG17Motor" method="GetPosition_Position"(reference=w635, error in=w648, "lChanID"=0) -> (error out=w646:errorcluster, "GetPosition_Position"=w640:sgl)  [unwired: 1 in, 2 out]
            n318 = invoke class="MG17Motor" method="GetPosition_Position"(reference=w634, error in=w646, "lChanID"=0) -> (error out=w645:errorcluster, "GetPosition_Position"=w639:sgl)  [unwired: 1 in, 2 out]
            n319 = property on="Experiment Region" class="Clust (strict)"(error in=w645) -> (error out=w644:errorcluster, "Value"=w643:T5)  [unwired: 1 in, 1 out]
            n320 = Bundle By Name(cluster=w643, "X Pos (mm)"=w639, "Y Pos (mm)"=w640, "Z Pos (mm)"=w641) -> (w642:T5)
            n321 = property on="Experiment Region" class="Clust (strict)"(error in=w644, "Value"=w642) -> (error out=w638:errorcluster)  [unwired: 1 in, 1 out]
          }
        }
      }
      event "GoToTopDisp": Value Change {
        n322 = event-data() -> ()  [unwired: 1 in, 1 out]
        n323 = property on="IsActive?" class="Bool (strict)"(error in=w663) -> (error out=w671:errorcluster, "Value"=w669:bool)  [unwired: 1 in, 1 out]
        n324 = property on="Motor Cruise Param" class="Clust (strict)"() -> ("Value"=w652:T11)  [unwired: 2 in, 2 out]
        n325 = Unbundle By Name(w652) -> ("X Acc (mm/s^2)"=w656:sgl, "X Vmax (mm/s)"=w655:sgl, "Y Acc (mm/s^2)"=w654:sgl, "Y Vmax (mm/s)"=w653:sgl, "Z Acc (mm/s^2)"=w658:sgl, "Z Vmax (mm/s)"=w657:sgl)
        n326 = property on="IsActive?" class="Bool (strict)"(error in=w671) -> (error out=w670:errorcluster, "Value"=w668:bool)  [unwired: 1 in, 1 out]
        n327 = property on="IsActive?" class="Bool (strict)"(error in=w670) -> (error out=w665:errorcluster, "Value"=w667:bool)  [unwired: 1 in, 1 out]
        n328 = Unbundle(w662) -> ("XMotorRef"=w661:refnum<k7>, "YMotorRef"=w660:refnum<k7>, "ZMotorRef"=w659:refnum<k7>)
        n329 = Compound Arithmetic op=AND(w669, w668, w667) -> (w666:bool)
        n330 = case shown="True" w666 {
          tunnel: w665 -> [w672 w692]
          tunnel: [w672 w688] -> w664
          tunnel: w661 -> [_ w715]
          tunnel: w660 -> [_ w700]
          tunnel: w659 -> [_ w687]
          tunnel: w658 -> [_ w678]
          tunnel: w657 -> [_ w677]
          tunnel: w656 -> [_ w676]
          tunnel: w655 -> [_ w675]
          tunnel: w654 -> [_ w674]
          tunnel: w653 -> [_ w673]
          frame False {
          }
          frame True {
            (unwired) 0 ("lChanID")
            n331 = invoke class="MG17Motor" method="StopImmediate"(reference=w715, error in=w692, "lChanID"=0) -> (reference out=w713:refnum<k7>, error out=w714:errorcluster, "lChanID"=w683:i32)  [unwired: 1 in, 1 out]
            n332 = invoke class="MG17Motor" method="StopImmediate"(reference=w700, error in=w692, "lChanID"=0) -> (reference out=w707:refnum<k7>, error out=w708:errorcluster, "lChanID"=w684:i32)  [unwired: 1 in, 1 out]
            n333 = invoke class="MG17Motor" method="StopImmediate"(reference=w687, error in=w692, "lChanID"=0) -> (reference out=w697:refnum<k7>, error out=w698:errorcluster, "lChanID"=w685:i32)  [unwired: 1 in, 1 out]
            n334 = property on="Top Dispenser" class="Clust (strict)"(error in=w692) -> ("Value"=w717:T5)  [unwired: 1 in, 2 out]
            n335 = invoke class="MG17Motor" method="SetVelParams"(reference=w697, error in=w698, "lChanID"=w685, "fMinVel"=sgl 0.0, "fAccn"=w678, "fMaxVel"=w677) -> (reference out=w696:refnum<k7>, error out=w695:errorcluster, "lChanID"=w694:i32)  [unwired: 1 in, 4 out]
            n336 = invoke class="MG17Motor" method="SetVelParams"(reference=w713, error in=w714, "lChanID"=w683, "fMinVel"=sgl 0.0, "fAccn"=w676, "fMaxVel"=w675) -> (reference out=w712:refnum<k7>, error out=w711:errorcluster, "lChanID"=w710:i32)  [unwired: 1 in, 4 out]
            n337 = invoke class="MG17Motor" method="SetVelParams"(reference=w707, error in=w708, "lChanID"=w684, "fMinVel"=sgl 0.0, "fAccn"=w674, "fMaxVel"=w673) -> (reference out=w705:refnum<k7>, error out=w704:errorcluster, "lChanID"=w703:i32)  [unwired: 1 in, 4 out]
            n338 = Unbundle By Name(w717) -> ("X Pos (mm)"=w681:sgl, "Y Pos (mm)"=w680:sgl, "Z Pos (mm)"=w679:sgl)
            n339 = invoke class="MG17Motor" method="MoveAbsoluteEx"(reference=w712, error in=w711, "lChanID"=w710, "fAbsPosCh1"=w681, "fAbsPosCh2"=w681, "bWait"=FALSE) -> (error out=w691:errorcluster)  [unwired: 1 in, 6 out]
            n340 = invoke class="MG17Motor" method="MoveAbsoluteEx"(reference=w705, error in=w704, "lChanID"=w703, "fAbsPosCh1"=w680, "fAbsPosCh2"=w680, "bWait"=FALSE) -> (error out=w690:errorcluster)  [unwired: 1 in, 6 out]
            n341 = invoke class="MG17Motor" method="MoveAbsoluteEx"(reference=w696, error in=w695, "lChanID"=w694, "fAbsPosCh1"=w679, "fAbsPosCh2"=w679, "bWait"=FALSE) -> (error out=w689:errorcluster)  [unwired: 1 in, 6 out]
            n342 = Merge Errors(w691, w690, w689) -> (w688:errorcluster)
          }
        }
      }
      event "GoToBottDisp": Value Change {
        n343 = event-data() -> ()  [unwired: 1 in, 1 out]
        n344 = property on="IsActive?" class="Bool (strict)"(error in=w729) -> (error out=w737:errorcluster, "Value"=w735:bool)  [unwired: 1 in, 1 out]
        n345 = property on="Motor Cruise Param" class="Clust (strict)"() -> ("Value"=w724:T11)  [unwired: 2 in, 2 out]
        n346 = Unbundle By Name(w724) -> ("X Acc (mm/s^2)"=w723:sgl, "X Vmax (mm/s)"=w722:sgl, "Y Acc (mm/s^2)"=w721:sgl, "Y Vmax (mm/s)"=w720:sgl, "Z Acc (mm/s^2)"=w719:sgl, "Z Vmax (mm/s)"=w718:sgl)
        n347 = property on="IsActive?" class="Bool (strict)"(error in=w737) -> (error out=w736:errorcluster, "Value"=w734:bool)  [unwired: 1 in, 1 out]
        n348 = property on="IsActive?" class="Bool (strict)"(error in=w736) -> (error out=w731:errorcluster, "Value"=w733:bool)  [unwired: 1 in, 1 out]
        n349 = Unbundle(w728) -> ("XMotorRef"=w727:refnum<k7>, "YMotorRef"=w726:refnum<k7>, "ZMotorRef"=w725:refnum<k7>)
        n350 = Compound Arithmetic op=AND(w735, w734, w733) -> (w732:bool)
        n351 = case shown="True" w732 {
          tunnel: w731 -> [w738 w758]
          tunnel: [w738 w754] -> w730
          tunnel: w727 -> [_ w781]
          tunnel: w726 -> [_ w766]
          tunnel: w725 -> [_ w753]
          tunnel: w723 -> [_ w744]
          tunnel: w722 -> [_ w743]
          tunnel: w721 -> [_ w742]
          tunnel: w720 -> [_ w741]
          tunnel: w719 -> [_ w740]
          tunnel: w718 -> [_ w739]
          frame False {
          }
          frame True {
            (unwired) 0 ("lChanID")
            n352 = invoke class="MG17Motor" method="StopImmediate"(reference=w781, error in=w758, "lChanID"=0) -> (reference out=w779:refnum<k7>, error out=w780:errorcluster, "lChanID"=w749:i32)  [unwired: 1 in, 1 out]
            n353 = invoke class="MG17Motor" method="StopImmediate"(reference=w766, error in=w758, "lChanID"=0) -> (reference out=w773:refnum<k7>, error out=w774:errorcluster, "lChanID"=w750:i32)  [unwired: 1 in, 1 out]
            n354 = invoke class="MG17Motor" method="StopImmediate"(reference=w753, error in=w758, "lChanID"=0) -> (reference out=w763:refnum<k7>, error out=w764:errorcluster, "lChanID"=w751:i32)  [unwired: 1 in, 1 out]
            n355 = property on="Bottom Dispenser" class="Clust (strict)"(error in=w758) -> ("Value"=w783:T5)  [unwired: 1 in, 2 out]
            n356 = invoke class="MG17Motor" method="SetVelParams"(reference=w779, error in=w780, "lChanID"=w749, "fMinVel"=sgl 0.0, "fAccn"=w744, "fMaxVel"=w743) -> (reference out=w778:refnum<k7>, error out=w777:errorcluster, "lChanID"=w776:i32)  [unwired: 1 in, 4 out]
            n357 = invoke class="MG17Motor" method="SetVelParams"(reference=w763, error in=w764, "lChanID"=w751, "fMinVel"=sgl 0.0, "fAccn"=w740, "fMaxVel"=w739) -> (reference out=w762:refnum<k7>, error out=w761:errorcluster, "lChanID"=w760:i32)  [unwired: 1 in, 4 out]
            n358 = invoke class="MG17Motor" method="SetVelParams"(reference=w773, error in=w774, "lChanID"=w750, "fMinVel"=sgl 0.0, "fAccn"=w742, "fMaxVel"=w741) -> (reference out=w771:refnum<k7>, error out=w770:errorcluster, "lChanID"=w769:i32)  [unwired: 1 in, 4 out]
            n359 = Unbundle By Name(w783) -> ("X Pos (mm)"=w747:sgl, "Y Pos (mm)"=w746:sgl, "Z Pos (mm)"=w745:sgl)
            n360 = invoke class="MG17Motor" method="MoveAbsoluteEx"(reference=w778, error in=w777, "lChanID"=w776, "fAbsPosCh1"=w747, "fAbsPosCh2"=w747, "bWait"=FALSE) -> (error out=w757:errorcluster)  [unwired: 1 in, 6 out]
            n361 = invoke class="MG17Motor" method="MoveAbsoluteEx"(reference=w771, error in=w770, "lChanID"=w769, "fAbsPosCh1"=w746, "fAbsPosCh2"=w746, "bWait"=FALSE) -> (error out=w756:errorcluster)  [unwired: 1 in, 6 out]
            n362 = invoke class="MG17Motor" method="MoveAbsoluteEx"(reference=w762, error in=w761, "lChanID"=w760, "fAbsPosCh1"=w745, "fAbsPosCh2"=w745, "bWait"=FALSE) -> (error out=w755:errorcluster)  [unwired: 1 in, 6 out]
            n363 = Merge Errors(w757, w756, w755) -> (w754:errorcluster)
          }
        }
      }
      event "GoToExpLoc": Value Change {
        n364 = event-data() -> ()  [unwired: 1 in, 1 out]
        n365 = property on="Motor Cruise Param" class="Clust (strict)"() -> ("Value"=w790:T11)  [unwired: 2 in, 2 out]
        n366 = property on="IsActive?" class="Bool (strict)"(error in=w795) -> (error out=w803:errorcluster, "Value"=w801:bool)  [unwired: 1 in, 1 out]
        n367 = Unbundle By Name(w790) -> ("X Acc (mm/s^2)"=w789:sgl, "X Vmax (mm/s)"=w788:sgl, "Y Acc (mm/s^2)"=w787:sgl, "Y Vmax (mm/s)"=w786:sgl, "Z Acc (mm/s^2)"=w785:sgl, "Z Vmax (mm/s)"=w784:sgl)
        n368 = property on="IsActive?" class="Bool (strict)"(error in=w803) -> (error out=w802:errorcluster, "Value"=w800:bool)  [unwired: 1 in, 1 out]
        n369 = property on="IsActive?" class="Bool (strict)"(error in=w802) -> (error out=w797:errorcluster, "Value"=w799:bool)  [unwired: 1 in, 1 out]
        n370 = Unbundle(w794) -> ("XMotorRef"=w793:refnum<k7>, "YMotorRef"=w792:refnum<k7>, "ZMotorRef"=w791:refnum<k7>)
        n371 = Compound Arithmetic op=AND(w801, w800, w799) -> (w798:bool)
        n372 = case shown="True" w798 {
          tunnel: w797 -> [w804 w824]
          tunnel: [w804 w820] -> w796
          tunnel: w793 -> [_ w847]
          tunnel: w792 -> [_ w832]
          tunnel: w791 -> [_ w819]
          tunnel: w789 -> [_ w810]
          tunnel: w788 -> [_ w809]
          tunnel: w787 -> [_ w808]
          tunnel: w786 -> [_ w807]
          tunnel: w785 -> [_ w806]
          tunnel: w784 -> [_ w805]
          frame False {
          }
          frame True {
            (unwired) 0 ("lChanID")
            n373 = invoke class="MG17Motor" method="StopImmediate"(reference=w847, error in=w824, "lChanID"=0) -> (reference out=w845:refnum<k7>, error out=w846:errorcluster, "lChanID"=w815:i32)  [unwired: 1 in, 1 out]
            n374 = invoke class="MG17Motor" method="StopImmediate"(reference=w832, error in=w824, "lChanID"=0) -> (reference out=w839:refnum<k7>, error out=w840:errorcluster, "lChanID"=w816:i32)  [unwired: 1 in, 1 out]
            n375 = invoke class="MG17Motor" method="StopImmediate"(reference=w819, error in=w824, "lChanID"=0) -> (reference out=w829:refnum<k7>, error out=w830:errorcluster, "lChanID"=w817:i32)  [unwired: 1 in, 1 out]
            n376 = property on="Experiment Region" class="Clust (strict)"(error in=w824) -> ("Value"=w849:T5)  [unwired: 1 in, 2 out]
            n377 = invoke class="MG17Motor" method="SetVelParams"(reference=w845, error in=w846, "lChanID"=w815, "fMinVel"=sgl 0.0, "fAccn"=w810, "fMaxVel"=w809) -> (reference out=w844:refnum<k7>, error out=w843:errorcluster, "lChanID"=w842:i32)  [unwired: 1 in, 4 out]
            n378 = invoke class="MG17Motor" method="SetVelParams"(reference=w829, error in=w830, "lChanID"=w817, "fMinVel"=sgl 0.0, "fAccn"=w806, "fMaxVel"=w805) -> (reference out=w828:refnum<k7>, error out=w827:errorcluster, "lChanID"=w826:i32)  [unwired: 1 in, 4 out]
            n379 = invoke class="MG17Motor" method="SetVelParams"(reference=w839, error in=w840, "lChanID"=w816, "fMinVel"=sgl 0.0, "fAccn"=w808, "fMaxVel"=w807) -> (reference out=w837:refnum<k7>, error out=w836:errorcluster, "lChanID"=w835:i32)  [unwired: 1 in, 4 out]
            n380 = Unbundle By Name(w849) -> ("X Pos (mm)"=w813:sgl, "Y Pos (mm)"=w812:sgl, "Z Pos (mm)"=w811:sgl)
            n381 = invoke class="MG17Motor" method="MoveAbsoluteEx"(reference=w844, error in=w843, "lChanID"=w842, "fAbsPosCh1"=w813, "fAbsPosCh2"=w813, "bWait"=FALSE) -> (error out=w823:errorcluster)  [unwired: 1 in, 6 out]
            n382 = invoke class="MG17Motor" method="MoveAbsoluteEx"(reference=w837, error in=w836, "lChanID"=w835, "fAbsPosCh1"=w812, "fAbsPosCh2"=w812, "bWait"=FALSE) -> (error out=w822:errorcluster)  [unwired: 1 in, 6 out]
            n383 = invoke class="MG17Motor" method="MoveAbsoluteEx"(reference=w828, error in=w827, "lChanID"=w826, "fAbsPosCh1"=w811, "fAbsPosCh2"=w811, "bWait"=FALSE) -> (error out=w821:errorcluster)  [unwired: 1 in, 6 out]
            n384 = Merge Errors(w823, w822, w821) -> (w820:errorcluster)
          }
        }
      }
      event "Steerable \nTrap\n(F12)": Value Change {
        # "Update the TTL signal to the shutter"
        n385 = event-data() -> ("NewVal"=w855:bool)  [unwired: 1 in]
        n386 = call-poly <vilib>:"DAQmx Create Virtual Channel.vi"("lines"=tag "PCI-6036E/port0/line0", "name to assign"="TrapA_TTL_Signal", "error in"=w853) -> ("task out"=w857:refnum<k21>, "error out"=w854:errorcluster)  [unwired: 11 in]
        n387 = call-poly <vilib>:"DAQmx Write.vi"("task/channels in"=w857, "data"=w855, "timeout"=10.0, "error in"=w854) -> ("task out"=w852:refnum<k21>, "error out"=w851:errorcluster)  [unwired: 9 in, 1 out]
        n388 = call <vilib>:"DAQmx Clear Task.vi"("task in"=w852, "error in"=w851) -> ("error out"=w850:errorcluster)  [unwired: 13 in]
      }
      event "Fixed\nTrap\n(F11)": Value Change {
        # "Update the TTL signal to the shutter"
        n389 = event-data() -> ("NewVal"=w865:bool)  [unwired: 1 in]
        n390 = call-poly <vilib>:"DAQmx Create Virtual Channel.vi"("lines"=tag "PCI-6036E/port0/line1", "name to assign"="TrapB_TTL_Signal", "error in"=w863) -> ("task out"=w867:refnum<k21>, "error out"=w864:errorcluster)  [unwired: 11 in]
        n391 = call-poly <vilib>:"DAQmx Write.vi"("task/channels in"=w867, "data"=w865, "timeout"=10.0, "error in"=w864) -> ("task out"=w862:refnum<k21>, "error out"=w861:errorcluster)  [unwired: 9 in, 1 out]
        n392 = call <vilib>:"DAQmx Clear Task.vi"("task in"=w862, "error in"=w861) -> ("error out"=w860:errorcluster)  [unwired: 13 in]
      }
      event "InterfaceSelector": Value Change {
        n393 = event-data() -> ("NewVal"=w872:T4)  [unwired: 1 in]
        n394 = case shown="\"Force-Extension (F4)\"" w872 {
          tunnel: [T1."BasicMode" T1."PassiveMode" T1."AcquireOffsetMode" T1."AcquireSpectrumMode" T1."Force-ExtensionMode"] -> w871
          frame "Basic Operation" {
          }
          frame "Passive Mode (F1)" {
            n395 = property on="IsPassiveModeActive?" class="Bool (strict)"("Value"=TRUE ("StopOffset")) -> ()  [unwired: 2 in, 2 out]
          }
          frame "Acquire Offset (F2)" {
            n396 = property on="IsOffsetModeActive?" class="Bool (strict)"("Value"=TRUE ("StopOffset")) -> ()  [unwired: 2 in, 2 out]
          }
          frame "Acquire Spectrum (F3)" {
          }
          frame "Force-Extension (F4)" {
            n397 = property on="IsForceExtActive?" class="Bool (strict)"("Value"=TRUE ("StopOffset")) -> ()  [unwired: 2 in, 2 out]
          }
        }
        "InstrumentMode" <- w871
      }
      event "BMSliderVert(V)": Value Change {
        # "Enforce Upper/Lower Limit for the axis voltage"
        # "X axis on the MadCityLabs controller, vertical bead motion"
        n398 = event-data() -> ()  [unwired: 1 in, 6 out]
        n399 = call-poly <vilib>:"DAQmx Create Virtual Channel.vi"("maximum value"=10.0 ("Maximum Value"), "minimum value"=0.0 ("Minimum Value"), "physical channels"=tag "PCI-6036E/ao1") -> ("task out"=w882:refnum<k21>, "error out"=w881:errorcluster)  [unwired: 11 in]
        n400 = In Range and Coerce(upper limit=10.0, x="BMSliderVert(V)", lower limit=0.0 ("upper limit")) -> (coerced(x)=w887:dbl)  [unwired: 1 out]
        n401 = call-poly <vilib>:"DAQmx Write.vi"("task/channels in"=w882, "data"=w887, "timeout"=10.0, "error in"=w881) -> ("task out"=w884:refnum<k21>, "error out"=w883:errorcluster)  [unwired: 9 in, 1 out]
        n402 = call <vilib>:"DAQmx Clear Task.vi"("task in"=w884, "error in"=w883) -> ()  [unwired: 13 in, 1 out]
      }
      event "BMHorizSlider(V)": Value Change {
        # "Enforce Upper/Lower Bounds"
        # "Y axis on the MadCityLabs controller corresponds to horizontall bead motion"
        n403 = event-data() -> ()  [unwired: 1 in, 6 out]
        n404 = call-poly <vilib>:"DAQmx Create Virtual Channel.vi"("maximum value"=10.0 ("Maximum Value"), "minimum value"=0.0 ("Minimum Value"), "physical channels"=tag "PCI-6036E/ao0") -> ("task out"=w895:refnum<k21>, "error out"=w894:errorcluster)  [unwired: 11 in]
        n405 = In Range and Coerce(upper limit=10.0, x="BMHorizSlider(V)", lower limit=0.0 ("upper limit")) -> (coerced(x)=w899:dbl)  [unwired: 1 out]
        n406 = call-poly <vilib>:"DAQmx Write.vi"("task/channels in"=w895, "data"=w899, "timeout"=10.0, "error in"=w894) -> ("task out"=w897:refnum<k21>, "error out"=w896:errorcluster)  [unwired: 9 in, 1 out]
        n407 = call <vilib>:"DAQmx Clear Task.vi"("task in"=w897, "error in"=w896) -> ()  [unwired: 13 in, 1 out]
      }
      event "StopOffset": Value Change {
        n408 = event-data() -> ("NewVal"=w905:bool)  [unwired: 1 in, 5 out]
        n409 = case shown="True" w905 {
          frame False {
          }
          frame True {
            n410 = flat-sequence {
              frame #0 {
                n411 = Not(x="StopOffset") -> (.not. x?=→"IsOffsetModeActive?":bool)
              }
              frame #1 {
                n412 = property on="InterfaceSelector" class="TabCtl (strict)"("Value"=T4."Basic Operation" ("InterfaceSelector")) -> ()  [unwired: 2 in, 2 out]
                n413 = property on="InstrumentMode" class="Enum (strict)"("Value"=T1."BasicMode" ("InstrumentMode")) -> ()  [unwired: 2 in, 2 out]
              }
            }
          }
        }
      }
      event "StopPassiveMode": Value Change {
        n414 = event-data() -> ("NewVal"=w910:bool)  [unwired: 1 in, 5 out]
        n415 = case shown="True" w910 {
          frame False {
          }
          frame True {
            n416 = flat-sequence {
              frame #0 {
                n417 = Not(x="StopPassiveMode") -> (.not. x?=→"IsPassiveModeActive?":bool)
              }
              frame #1 {
                n418 = property on="InterfaceSelector" class="TabCtl (strict)"("Value"=T4."Basic Operation" ("InterfaceSelector")) -> ()  [unwired: 2 in, 2 out]
                n419 = property on="InstrumentMode" class="Enum (strict)"("Value"=T1."BasicMode" ("InstrumentMode")) -> ()  [unwired: 2 in, 2 out]
              }
            }
          }
        }
      }
      event "StopForceExtension": Value Change {
        n420 = event-data() -> ("NewVal"=w915:bool)  [unwired: 1 in, 5 out]
        n421 = case shown="True" w915 {
          frame False {
          }
          frame True {
            n422 = flat-sequence {
              frame #0 {
                n423 = Not(x="StopForceExtension") -> (.not. x?=→"IsForceExtActive?":bool)
              }
              frame #1 {
                n424 = property on="InterfaceSelector" class="TabCtl (strict)"("Value"=T4."Basic Operation" ("InterfaceSelector")) -> ()  [unwired: 2 in, 2 out]
                n425 = property on="InstrumentMode" class="Enum (strict)"("Value"=T1."BasicMode" ("InstrumentMode")) -> ()  [unwired: 2 in, 2 out]
              }
            }
          }
        }
      }
      event "Stop": Value Change {
        n426 = event-data() -> ()  [unwired: 1 in, 1 out]
        n427 = property on="InstrumentMode" class="Enum (strict)"("Value"=T1."Shutdown") -> ()  [unwired: 2 in, 2 out]
      }
    }
  }
  n428 = while {
    shift-right: [w924] -> _
    shift-left: T1."InitializeJoystick" -> [w923]
    shift-right: [w941] -> _
    shift-left: _ -> [w934]
    shift-right: [w938] -> w5
    shift-left: _ -> [w940]
    shift-right: [w939] -> _
    shift-left: _ -> [w937]
    shift-right: [w936] -> _
    shift-left: _ -> [w935]
    shift-right: [w933] -> _
    shift-left: _ -> [w930]
    shift-right: [w931] -> _
    shift-left: _ -> [w932]
    stop <- w925 stop-if-true
    # "Motor Control Loop"
    # ">Joystick Offset>"
    # ">RelJoyPos>"
    # ">XYZ Motor Ref>"
    # ">Error>"
    # ">Joystick Task ID>"
    # ">Joystick Buttons>"
    n429 = control-ref of="Steerable \nTrap\n(F12)"() -> (w927:refnum<vi>)
    n430 = control-ref of="Fixed\nTrap\n(F11)"() -> (w928:refnum<vi>)
    n431 = Bundle("Steerable \nTrap\n(F12)"=w927, "Fixed\nTrap\n(F11)"=w928) -> (w926:T24)  [unwired: 1 in]
    n432 = Wait (ms)(milliseconds to wait="MotorLoopDelay") -> ()  [unwired: 1 out]
    n433 = case shown="\"InitializeJoystick\"" w923 {
      tunnel: [w970 _ w1058 w1148 w1155 w1162 w1169 _] -> w941
      tunnel: [T1."InitializeMotors" w974 w1042 w1152 w1159 w1166 w1173 w1192] -> w924
      tunnel: w940 -> [_ w1023 w1060 w1151 w1158 w1165 w1172 w1177]
      tunnel: [w969 _ w1059 w1146 w1153 w1160 w1167 _] -> w939
      tunnel: [w945 w1022 w1051 w1151 w1158 w1165 w1172 w1174] -> w938
      tunnel: w937 -> [_ _ w1061 w1146 w1153 w1160 w1167 w1176]
      tunnel: [_ _ w1045 w1147 w1154 w1161 w1168 _] -> w936
      tunnel: w935 -> [_ _ w1044 w1147 w1154 w1161 w1168 _]
      tunnel: w934 -> [_ _ w1056 w1148 w1155 w1162 w1169 _]
      tunnel: [_ _ _ _ _ _ _ TRUE ("status")] -> w925
      tunnel: [_ w1021 w1050 w1150 w1157 w1164 w1171 _] -> w933
      tunnel: w930 -> [_ _ w1050 w1150 w1157 w1164 w1171 w1178]
      tunnel: [_ _ w1048 w1149 w1156 w1163 w1170 _] -> w931
      tunnel: w932 -> [_ _ w1057 w1149 w1156 w1163 w1170 _]
      tunnel: w926 -> [w960 _ w1043 _ _ _ _ _]
      frame "InitializeJoystick" {
        # "Initialize Joystick and Shutter Controls"
        n434 = property on="JoystOffset" class="Clust (strict)"() -> ("Value"=w968:T2)  [unwired: 2 in, 2 out]
        n435 = Bundle By Name(cluster=w968, "XOffset"=-99999, "YOffset"=-99999, "ZOffset"=-99999) -> (w970:T2)
        n436 = Unbundle(w960) -> ("Steerable \nTrap\n(F12)"=w949:refnum<vi>, "Fixed\nTrap\n(F11)"=w948:refnum<vi>)
        n437 = call <vilib>:"Initialize Joystick.vi"() -> ("error out"=w950:errorcluster, "device ID"=w969:refnum<k1>)  [unwired: 10 in]
        n438 = call-poly <vilib>:"DAQmx Create Virtual Channel.vi"("lines"=tag "PCI-6036E/port0/line1", "name to assign"="TrapB_TTL_Signal", "error in"=w950) -> ("task out"=w956:refnum<k21>, "error out"=w958:errorcluster)  [unwired: 11 in]
        n439 = call-poly <vilib>:"DAQmx Create Virtual Channel.vi"("lines"=tag "PCI-6036E/port0/line0", "name to assign"="TrapA_TTL_Signal", "error in"=w950) -> ("task out"=w965:refnum<k21>, "error out"=w967:errorcluster)  [unwired: 11 in]
        n440 = call-poly <vilib>:"DAQmx Read.vi"("task/channels in"=w956, "timeout"=10.0, "error in"=w958) -> ("task out"=w952:refnum<k21>, "data"=w943:bool, "error out"=w953:errorcluster)  [unwired: 10 in]
        n441 = call-poly <vilib>:"DAQmx Read.vi"("task/channels in"=w965, "timeout"=10.0, "error in"=w967) -> ("task out"=w961:refnum<k21>, "data"=w944:bool, "error out"=w962:errorcluster)  [unwired: 10 in]
        n442 = property class="Bool (strict)"(reference=w949, error in=w962, "Value"=w944) -> (error out=w959:errorcluster)  [unwired: 1 out]
        n443 = property class="Bool (strict)"(reference=w948, error in=w953, "Value"=w943) -> (error out=w951:errorcluster)  [unwired: 1 out]
        n444 = call <vilib>:"DAQmx Clear Task.vi"("task in"=w952, "error in"=w951) -> ("error out"=w946:errorcluster)  [unwired: 13 in]
        n445 = call <vilib>:"DAQmx Clear Task.vi"("task in"=w961, "error in"=w959) -> ("error out"=w947:errorcluster)  [unwired: 13 in]
        n446 = Merge Errors(w947, w946) -> (w945:errorcluster)
      }
      frame "InitializeMotors" {
        w974 = T1."BasicMode"
        w1027 = 83829794  # Z Axis Controller ID
        w1033 = 83829822  # Y Axis Controller ID
        w1039 = 83829798  # X Axis Controller ID
        n447 = property on="IsActive?" class="Bool (strict)"(error in=w1023, "Value"=FALSE ("IsYMotorActive?")) -> (error out=w1034:errorcluster)  [unwired: 1 in, 1 out]
        n448 = property on="IsActive?" class="Bool (strict)"(error in=w1023, "Value"=FALSE ("IsYMotorActive?")) -> (error out=w1040:errorcluster)  [unwired: 1 in, 1 out]
        n449 = property on="IsActive?" class="Bool (strict)"(error in=w1023, "Value"=FALSE ("IsYMotorActive?")) -> (error out=w1028:errorcluster)  [unwired: 1 in, 1 out]
        n450 = call "s_InitializeMotor.vi"("Error In"=w1034, "Servo Controller  ID"=w1033, "Motor Reference In"="YMotorRef") -> ("Error Out"=w1035:errorcluster, "Motor Reference"=w1016:refnum<k7>)
        n451 = call "s_InitializeMotor.vi"("Error In"=w1040, "Servo Controller  ID"=w1039, "Motor Reference In"="XMotorRef") -> ("Error Out"=w1041:errorcluster, "Motor Reference"=w1020:refnum<k7>)
        n452 = call "s_InitializeMotor.vi"("Error In"=w1028, "Servo Controller  ID"=w1027, "Motor Reference In"="ZMotorRef") -> ("Error Out"=w1029:errorcluster, "Motor Reference"=w1013:refnum<k7>)
        n453 = property on="IsActive?" class="Bool (strict)"(error in=w1035, "Value"=TRUE ("IsYMotorActive?")) -> (error out=w1015:errorcluster)  [unwired: 1 in, 1 out]
        n454 = Unbundle By Name("Motor Limits") -> ("XMin"=w980:sgl, "XMax"=w979:sgl, "YMin"=w978:sgl, "YMax"=w977:sgl, "ZMin"=w976:sgl, "ZMax"=w975:sgl)
        n455 = property on="IsActive?" class="Bool (strict)"(error in=w1041, "Value"=TRUE ("IsYMotorActive?")) -> (error out=w1018:errorcluster)  [unwired: 1 in, 1 out]
        n456 = property on="IsActive?" class="Bool (strict)"(error in=w1029, "Value"=TRUE ("IsYMotorActive?")) -> (error out=w1012:errorcluster)  [unwired: 1 in, 1 out]
        n457 = invoke class="MG17Motor" method="SetStageAxisInfo"(reference=w1020, error in=w1018, "lChanID"=0, "fMinPos"=w980, "fMaxPos"=w979, "lUnits"=1, "fPitch"=sgl 1.0, "lDirSense"=0) -> (reference out=w1011:refnum<k7>, error out=w1010:errorcluster, "lChanID"=w1009:i32)  [unwired: 1 in, 6 out]
        n458 = invoke class="MG17Motor" method="SetStageAxisInfo"(reference=w1016, error in=w1015, "lChanID"=0, "fMinPos"=w978, "fMaxPos"=w977, "lUnits"=1, "fPitch"=sgl 1.0, "lDirSense"=0) -> (reference out=w1003:refnum<k7>, error out=w1002:errorcluster, "lChanID"=w1001:i32)  [unwired: 1 in, 6 out]
        n459 = invoke class="MG17Motor" method="SetStageAxisInfo"(reference=w1013, error in=w1012, "lChanID"=0, "fMinPos"=w976, "fMaxPos"=w975, "lUnits"=1, "fPitch"=sgl 1.0, "lDirSense"=0) -> (reference out=w998:refnum<k7>, error out=w997:errorcluster, "lChanID"=w996:i32)  [unwired: 1 in, 6 out]
        n460 = invoke class="MG17Motor" method="GetPosition_Position"(reference=w1003, error in=w1002, "lChanID"=w1001) -> (reference out=w995:refnum<k7>, error out=w1005:errorcluster, "GetPosition_Position"=w1004:sgl)  [unwired: 1 in, 1 out]
        n461 = invoke class="MG17Motor" method="GetPosition_Position"(reference=w998, error in=w997, "lChanID"=w996) -> (reference out=w994:refnum<k7>, error out=w1000:errorcluster, "GetPosition_Position"=w999:sgl)  [unwired: 1 in, 1 out]
        n462 = invoke class="MG17Motor" method="GetPosition_Position"(reference=w1011, error in=w1010, "lChanID"=w1009) -> (reference out=w1008:refnum<k7>, error out=w1007:errorcluster, "GetPosition_Position"=w1006:sgl)  [unwired: 1 in, 1 out]
        n463 = property on="Pos (mm)" class="DigNum (strict)"(error in=w1005, "Value"=w1004) -> (error out=w993:errorcluster)  [unwired: 1 in, 1 out]
        n464 = property on="Pos (mm)" class="DigNum (strict)"(error in=w1000, "Value"=w999) -> (error out=w991:errorcluster)  [unwired: 1 in, 1 out]
        n465 = property on="Pos (mm)" class="DigNum (strict)"(error in=w1007, "Value"=w1006) -> (error out=w992:errorcluster)  [unwired: 1 in, 1 out]
        n466 = Bundle("Motor Reference"=w1008, "Motor Reference"=w995, "Motor Reference"=w994) -> (w1021:T25)  [unwired: 1 in]
        n467 = Merge Errors(w992, w993, w991) -> (w1022:errorcluster)
        n468 = property on="InstrumentMode" class="Enum (strict)"("Value"=w974) -> ()  [unwired: 2 in, 2 out]
      }
      frame "BasicMode" {
        n469 = call-poly <vilib>:"Acquire Input Data.vi"("device ID"=w1061, "error in (no error)"=w1060) -> ("device ID"=w1059:refnum<k1>, "axis info"=w1055:T26, "button info"=w1045:T27, "error out"=w1047:errorcluster)  [unwired: 13 in, 1 out]
        n470 = call "j_GetJoystickSignal.vi"("RelJoyPos In"=w1057, "NewJoystButtInfo"=w1045, "NewJoystAxisInfo"=w1055, "OldJoystButtInfo"=w1044, "OldJoystickOffset"=w1056) -> ("MoveZ"=→"Move Z":bool, "MoveXY"=→"Move XY":bool, "Joystick Offset"=w1058:T2, "RelJoyPos"=w1052:T3, "TalkToMotors?"=w1049:bool)
        n471 = call "s_TurnTrapsOnOffWithJoystick.vi"("Error In"=w1047, "Shutter Control Reference Cluster"=w1043, "NewJoystButtInfo"=w1045, "OldJoystButtInfo"=w1044) -> ("Error Out"=w1046:errorcluster)  [unwired: 7 in]
        n472 = case shown="True" w1049 {
          tunnel: w1052 -> [w1099 w1103]
          tunnel: [w1088 w1120] -> w1051
          tunnel: w1050 -> [w1098 w1106]
          tunnel: w1046 -> [w1072 w1105]
          tunnel: [w1099 w1103] -> w1048
          frame False {
            # "Just Update Motor Position and Vel"
            n473 = Unbundle(w1098) -> ("Motor Reference"=w1097:refnum<k7>, "Motor Reference"=w1090:refnum<k7>, "Motor Reference"=w1089:refnum<k7>)
            n474 = property on="Pos (mm)" class="DigNum (strict)"(error in=w1072) -> (error out=w1080:errorcluster, "Value"=w1077:sgl)  [unwired: 1 in, 1 out]
            n475 = property on="Pos (mm)" class="DigNum (strict)"(error in=w1072) -> (error out=w1073:errorcluster, "Value"=w1070:sgl)  [unwired: 1 in, 1 out]
            n476 = property on="Pos (mm)" class="DigNum (strict)"(error in=w1072) -> (error out=w1081:errorcluster, "Value"=w1086:sgl)  [unwired: 1 in, 1 out]
            n477 = invoke class="MG17Motor" method="GetPosition_Position"(reference=w1090, error in=w1080, "lChanID"=0) -> (error out=w1093:errorcluster, "GetPosition_Position"=w1078:sgl)  [unwired: 1 in, 2 out]
            n478 = invoke class="MG17Motor" method="GetPosition_Position"(reference=w1089, error in=w1073, "lChanID"=0) -> (error out=w1091:errorcluster, "GetPosition_Position"=w1069:sgl)  [unwired: 1 in, 2 out]
            n479 = property on="MotorLoopDelay" class="DigNum (strict)"() -> ("Value"=w1065:u32)  [unwired: 2 in, 2 out]
            n480 = invoke class="MG17Motor" method="GetPosition_Position"(reference=w1097, error in=w1081, "lChanID"=0) -> (error out=w1095:errorcluster, "GetPosition_Position"=w1087:sgl)  [unwired: 1 in, 2 out]
            n481 = To Single Precision Float(number=w1065) -> (single precision float=w1064:sgl)
            n482 = Subtract(x=w1087, y=w1086) -> (x-y=w1085:sgl)
            n483 = property on="Pos (mm)" class="DigNum (strict)"(error in=w1093, "Value"=w1078) -> (error out=w1076:errorcluster)  [unwired: 1 in, 1 out]
            n484 = Subtract(x=w1078, y=w1077) -> (x-y=w1079:sgl)
            n485 = Subtract(x=w1069, y=w1070) -> (x-y=w1071:sgl)
            n486 = property on="Pos (mm)" class="DigNum (strict)"(error in=w1091, "Value"=w1069) -> (error out=w1068:errorcluster)  [unwired: 1 in, 1 out]
            n487 = property on="Pos (mm)" class="DigNum (strict)"(error in=w1095, "Value"=w1087) -> (error out=w1083:errorcluster)  [unwired: 1 in, 1 out]
            n488 = Divide(x=w1064, y=sgl 1000.0) -> (x/y=w1062:sgl)
            n489 = Divide(x=w1085, y=w1062) -> (x/y=w1084:sgl)
            n490 = Divide(x=w1079, y=w1062) -> (x/y=w1075:sgl)
            n491 = Divide(x=w1071, y=w1062) -> (x/y=w1067:sgl)
            n492 = property on="Vel (mm/s)" class="DigNum (strict)"(error in=w1083, "Value"=w1084) -> (error out=w1082:errorcluster)  [unwired: 1 in, 1 out]
            n493 = property on="Vel (mm/s)" class="DigNum (strict)"(error in=w1076, "Value"=w1075) -> (error out=w1074:errorcluster)  [unwired: 1 in, 1 out]
            n494 = property on="Vel (mm/s)" class="DigNum (strict)"(error in=w1068, "Value"=w1067) -> (error out=w1066:errorcluster)  [unwired: 1 in, 1 out]
            n495 = Merge Errors(w1082, w1074, w1066) -> (w1088:errorcluster)
          }
          frame True {
            # ">ZMotRef>"
            # ">YMotRef>"
            # ">XMotRef>"
            n496 = Unbundle By Name(w1103) -> ("XRelPos"=w1136:i32, "YRelPos"=w1122:i32, "ZRelPos"=w1107:i32)
            n497 = Unbundle(w1106) -> ("Motor Reference"=w1102:refnum<k7>, "Motor Reference"=w1101:refnum<k7>, "Motor Reference"=w1100:refnum<k7>)
            n498 = property on="Direction" class="DigNum (strict)"(error in=w1105) -> (error out=w1135:errorcluster, "Value"=w1134:i32)  [unwired: 1 in, 1 out]
            n499 = property on="Direction" class="DigNum (strict)"(error in=w1105) -> (error out=w1125:errorcluster, "Value"=w1124:i32)  [unwired: 1 in, 1 out]
            n500 = property on="Direction" class="DigNum (strict)"(error in=w1105) -> (error out=w1110:errorcluster, "Value"=w1109:i32)  [unwired: 1 in, 1 out]
            n501 = property on="Move Z" class="Bool (strict)"(error in=w1110) -> (error out=w1118:errorcluster, "Value"=w1117:bool)  [unwired: 1 in, 1 out]
            n502 = property on="Move XY" class="Bool (strict)"(error in=w1135) -> (error out=w1144:errorcluster, "Value"=w1143:bool)  [unwired: 1 in, 1 out]
            n503 = property on="Move XY" class="Bool (strict)"(error in=w1125) -> (error out=w1133:errorcluster, "Value"=w1132:bool)  [unwired: 1 in, 1 out]
            n504 = call "j_MotorExecute.vi"("MoveChamber?"=w1143, "Axis Motor Settings"="X Motor Settings", "Error In"=w1144, "JoystRelPos"=w1136, "Motor's Old Direction"=w1134, "Motor Reference In"=w1102) -> ("Error Out"=w1139:errorcluster, "Motor Position (mm)"=w1138:sgl, "Motor's New Direction"=w1137:i32, "Motor Velocity (mm/s)"=w1140:sgl)  [unwired: 1 out]
            n505 = call "j_MotorExecute.vi"("MoveChamber?"=w1132, "Axis Motor Settings"="Y Motor Settings", "Error In"=w1133, "JoystRelPos"=w1122, "Motor's Old Direction"=w1124, "Motor Reference In"=w1101) -> ("Error Out"=w1128:errorcluster, "Motor Position (mm)"=w1127:sgl, "Motor's New Direction"=w1126:i32, "Motor Velocity (mm/s)"=w1129:sgl)  [unwired: 1 out]
            n506 = call "j_MotorExecute.vi"("MoveChamber?"=w1117, "Axis Motor Settings"="Z Motor Settings", "Error In"=w1118, "JoystRelPos"=w1107, "Motor's Old Direction"=w1109, "Motor Reference In"=w1100) -> ("Error Out"=w1113:errorcluster, "Motor Position (mm)"=w1112:sgl, "Motor's New Direction"=w1111:i32, "Motor Velocity (mm/s)"=w1114:sgl)  [unwired: 1 out]
            n507 = property on="Pos (mm)" class="DigNum (strict)"(error in=w1139, "Value"=w1138) -> (error out=w1141:errorcluster)  [unwired: 1 in, 1 out]
            n508 = property on="Pos (mm)" class="DigNum (strict)"(error in=w1128, "Value"=w1127) -> (error out=w1130:errorcluster)  [unwired: 1 in, 1 out]
            n509 = property on="Pos (mm)" class="DigNum (strict)"(error in=w1113, "Value"=w1112) -> (error out=w1115:errorcluster)  [unwired: 1 in, 1 out]
            n510 = property on="Vel (mm/s)" class="DigNum (strict)"(error in=w1141, "Value"=w1140) -> (error out=w1142:errorcluster)  [unwired: 1 in, 1 out]
            n511 = property on="Vel (mm/s)" class="DigNum (strict)"(error in=w1130, "Value"=w1129) -> (error out=w1131:errorcluster)  [unwired: 1 in, 1 out]
            n512 = property on="Vel (mm/s)" class="DigNum (strict)"(error in=w1115, "Value"=w1114) -> (error out=w1116:errorcluster)  [unwired: 1 in, 1 out]
            n513 = property on="Direction" class="DigNum (strict)"(error in=w1131, "Value"=w1126) -> (error out=w1119:errorcluster)  [unwired: 1 in, 1 out]
            n514 = property on="Direction" class="DigNum (strict)"(error in=w1142, "Value"=w1137) -> (error out=w1121:errorcluster)  [unwired: 1 in, 1 out]
            n515 = property on="Direction" class="DigNum (strict)"(error in=w1116, "Value"=w1111) -> (error out=w1104:errorcluster)  [unwired: 1 in, 1 out]
            n516 = Merge Errors(w1121, w1119, w1104) -> (w1120:errorcluster)
          }
        }
        n517 = property on="InstrumentMode" class="Enum (strict)"() -> ("Value"=w1042:T1)  [unwired: 2 in, 2 out]
      }
      frame "PassiveMode" {
        n518 = property on="InstrumentMode" class="Enum (strict)"() -> ("Value"=w1152:T1)  [unwired: 2 in, 2 out]
      }
      frame "AcquireOffsetMode" {
        n519 = property on="InstrumentMode" class="Enum (strict)"() -> ("Value"=w1159:T1)  [unwired: 2 in, 2 out]
      }
      frame "AcquireSpectrumMode" {
        n520 = property on="InstrumentMode" class="Enum (strict)"() -> ("Value"=w1166:T1)  [unwired: 2 in, 2 out]
      }
      frame "Force-ExtensionMode" {
        n521 = property on="InstrumentMode" class="Enum (strict)"() -> ("Value"=w1173:T1)  [unwired: 2 in, 2 out]
      }
      frame "Shutdown" {
        n522 = call-poly <vilib>:"Close Input Device.vi"("error in (no error)"=w1177, "device ID"=w1176) -> ("error out"=w1185:errorcluster)  [unwired: 8 in]
        n523 = Unbundle(w1178) -> ("Motor Reference"=w1181:refnum<k7>, "Motor Reference"=w1180:refnum<k7>, "Motor Reference"=w1179:refnum<k7>)
        n524 = call "s_CloseMotor.vi"("Error In"=w1185, "Motor Reference In"=w1181) -> ("Error Out"=w1190:errorcluster)
        n525 = call "s_CloseMotor.vi"("Error In"=w1185, "Motor Reference In"=w1180) -> ("Error Out"=w1188:errorcluster)
        n526 = call "s_CloseMotor.vi"("Error In"=w1185, "Motor Reference In"=w1179) -> ("Error Out"=w1186:errorcluster)
        n527 = property on="IsActive?" class="Bool (strict)"(error in=w1190, "Value"=FALSE ("IsYMotorActive?")) -> (error out=w1184:errorcluster)  [unwired: 1 in, 1 out]
        n528 = property on="IsActive?" class="Bool (strict)"(error in=w1188, "Value"=FALSE ("IsYMotorActive?")) -> (error out=w1183:errorcluster)  [unwired: 1 in, 1 out]
        n529 = property on="IsActive?" class="Bool (strict)"(error in=w1186, "Value"=FALSE ("IsYMotorActive?")) -> (error out=w1182:errorcluster)  [unwired: 1 in, 1 out]
        n530 = Merge Errors(w1184, w1183, w1182) -> (w1175:errorcluster)
        n531 = property on="InstrumentMode" class="Enum (strict)"(error in=w1175) -> (error out=w1174:errorcluster, "Value"=w1192:T1)  [unwired: 1 in, 1 out]
      }
    }
  }
  n532 = Merge Errors(w1, w5, w7) -> (w3:errorcluster)
  n533 = call <vilib>:"General Error Handler.vi"("type of dialog (OK msg:1)"=w2, "error in (no error)"=w3) -> ()  [unwired: 9 in, 5 out]
